vi "Farming robot v2.vi"() -> ()   [LabVIEW 2021]
uses:
  <vilib>/myRIO/Instrument Drivers/Onboard IO/DIO/typedefs/DIO Reference.ctl
  <vilib>/myRIO/Common/Instrument Driver Framework/Utilities/typedefs/myRIO Generic Hardware Reference.ctl
  <vilib>/myRIO/Common/Instrument Driver Framework/Utilities/typedefs/Hardware Version Enum.ctl
  <vilib>/myRIO/Common/Instrument Driver Framework/Utilities/typedefs/myRIO v1.0 Reference.ctl
  <vilib>/myRIO/Common/Instrument Driver Framework/Utilities/typedefs/Generic FPGA Reference.ctl
  <vilib>/myRIO/Common/Instrument Driver Framework/myRIO v1.0/DIO/typedefs/DIO Channels List.ctl
  <vilib>/myRIO/Common/Instrument Driver Framework/myRIO v1.0/DIO/typedefs/DIO Channels Enum.ctl
  <vilib>/userDefined/High Color/nirio_resource_hc.ctl
  <vilib>/myRIO/Instrument Drivers/Onboard IO/PWM/typedefs/PWM Reference.ctl
  <vilib>/myRIO/Common/Instrument Driver Framework/myRIO v1.0/PWM/typedefs/PWM Channels Enum.ctl
  <vilib>/myRIO/Instrument Drivers/Onboard IO/PWM/typedefs/PWM Configuration.ctl
  <vilib>/myRIO/Instrument Drivers/Onboard Devices/Accelerometer/typedefs/Accelerometer Reference.ctl
  <vilib>/myRIO/Common/Instrument Driver Framework/myRIO v1.0/Accelerometer/typedefs/Accelerometer Channels List.ctl
  <vilib>/myRIO/Common/Instrument Driver Framework/myRIO v1.0/Accelerometer/typedefs/Accelerometer Channels Enum.ctl
  <vilib>/myRIO/Common/Instrument Driver Framework/Utilities/vis/Is FPGA Ref Available.vi
  <vilib>/myRIO/Common/Instrument Driver Framework/myRIO v1.0/DIO/vis/myRIO v1.1 Open DIO.vi
  <vilib>/myRIO/Instrument Drivers/Onboard IO/DIO/vis/Write.vi
  <vilib>/myRIO/Common/Instrument Driver Framework/myRIO v1.0/Accelerometer/vis/myRIO v1.1 Open Accelerometer.vi
  <vilib>/myRIO/Instrument Drivers/Onboard Devices/Accelerometer/vis/Read.vi
  <vilib>/myRIO/Common/Instrument Driver Framework/myRIO v1.0/PWM/vis/myRIO v1.1 Open PWM.vi
  <vilib>/myRIO/Instrument Drivers/Onboard IO/PWM/vis/Set Duty Cycle and Frequency.vi
  <vilib>/myRIO/Common/Instrument Driver Framework/Utilities/vis/Validate Channels.vi
  <vilib>/myRIO/Common/Instrument Driver Framework/myRIO v1.0/DIO/vis/myRIO v1.0 Reserve DIO.vi
  <vilib>/myRIO/Common/Instrument Driver Framework/myRIO v1.0/Accelerometer/vis/myRIO v1.0 Reserve Accelerometer.vi
  <vilib>/myRIO/Common/Instrument Driver Framework/myRIO v1.0/PWM/vis/myRIO v1.0 Reserve PWM.vi
  <vilib>/myRIO/Common/Instrument Driver Framework/myRIO v1.0/Resource Manager/vis/myRIO v1.0 Reserve Channel List.vi
  <vilib>/myRIO/Common/Instrument Driver Framework/myRIO v1.0/DIO/vis/myRIO v1.0 Build MUX Configuration DIO.vi
  <vilib>/myRIO/Common/Instrument Driver Framework/myRIO v1.0/Accelerometer/vis/myRIO v1.0 Build MUX Configuration Accelerometer.vi
  <vilib>/myRIO/Common/Instrument Driver Framework/myRIO v1.0/PWM/vis/myRIO v1.0 Build MUX Configuration PWM.vi
  <vilib>/myRIO/Common/Instrument Driver Framework/myRIO v1.0/Resource Manager/vis/myRIO v1.0 Reserve Channel.vi
  <vilib>/myRIO/Common/Instrument Driver Framework/myRIO v1.0/Resource Manager/vis/myRIO v1.0 Unreserve Channel.vi
  <vilib>/myRIO/Common/Instrument Driver Framework/myRIO v1.0/Resource Manager/vis/myRIO v1.0 Create Configuration List.vi
  <vilib>/myRIO/Common/Instrument Driver Framework/myRIO v1.0/Resource Manager/vis/myRIO v1.0 Build Mutex Name.vi
  <vilib>/Utility/VariantDataType/GetNumericInfo.vi
  <vilib>/Utility/error.llb/Error Cluster From Error Code.vi
  <vilib>/myRIO/Common/Instrument Driver Framework/myRIO v1.0/myRIO v1.1 Open.vi
  <vilib>/myRIO/Common/Instrument Driver Framework/Utilities/vis/IO Manager.vi
  <vilib>/myRIO/Common/Instrument Driver Framework/Utilities/vis/Configuration Manager.vi
  <vilib>/myRIO/Common/Instrument Driver Framework/myRIO v1.0/Resource Manager/vis/myRIO v1.0 Configure IO.vi
  <vilib>/myRIO/Common/Instrument Driver Framework/myRIO v1.0/myRIO v1.0 Close.vi
  <vilib>/myRIO/Common/Instrument Driver Framework/myRIO v1.0/DIO/vis/myRIO v1.0 Write DIO.vi
  <vilib>/myRIO/Common/Instrument Driver Framework/myRIO v1.0/PWM/vis/myRIO v1.0 Write PWM.vi
  <vilib>/myRIO/Common/Instrument Driver Framework/myRIO v1.0/Accelerometer/vis/myRIO v1.0 Get Scaling Constant Accelerometer.vi
  <vilib>/myRIO/Common/Instrument Driver Framework/myRIO v1.0/Accelerometer/vis/myRIO v1.0 Read Accelerometer.vi
  <vilib>/myRIO/Express VI/Onboard Devices/LED/LED Express VI.xnode
  <vilib>/myRIO/Instrument Drivers/Onboard IO/DIO/vis/myRIO DIO Open.xnode
  <vilib>/myRIO/Express VI/Onboard IO/DO/DO Express VI.xnode
  <vilib>/myRIO/Express VI/Onboard IO/PWM/PWM Express VI.xnode
  <vilib>/myRIO/Instrument Drivers/Onboard IO/PWM/vis/myRIO PWM Open.xnode
  <vilib>/myRIO/Express VI/Onboard Devices/Accelerometer/Accelerometer Express VI.xnode
  <vilib>/myRIO/Instrument Drivers/Onboard Devices/Accelerometer/vis/myRIO Accelerometer Open.xnode
  <vilib>/myRIO/Instrument Drivers/Onboard IO/DIO/DIO.lvlib
  <vilib>/myRIO/Instrument Drivers/Onboard Devices/Accelerometer/Accelerometer.lvlib
  <vilib>/myRIO/Instrument Drivers/Onboard IO/PWM/PWM.lvlib
  <vilib>/Analysis/NI_AALPro.lvlib
panel:
  out "pulse width 2":dbl
  out "Angle 2":dbl
  out "State":T1(ring)
  out "pulse width 1":dbl
  out "Angle 1":dbl
  in  "Start Farming":bool
  out "Watering":bool
  out "Seeding\nUp":bool
  out "Seeding\nDown":bool
  out "Switching\nMode":bool
  out "Drill Up":bool
  out "Drill Down":bool
  out "Intialize":bool
  out "Message":string
  in  "stop":bool
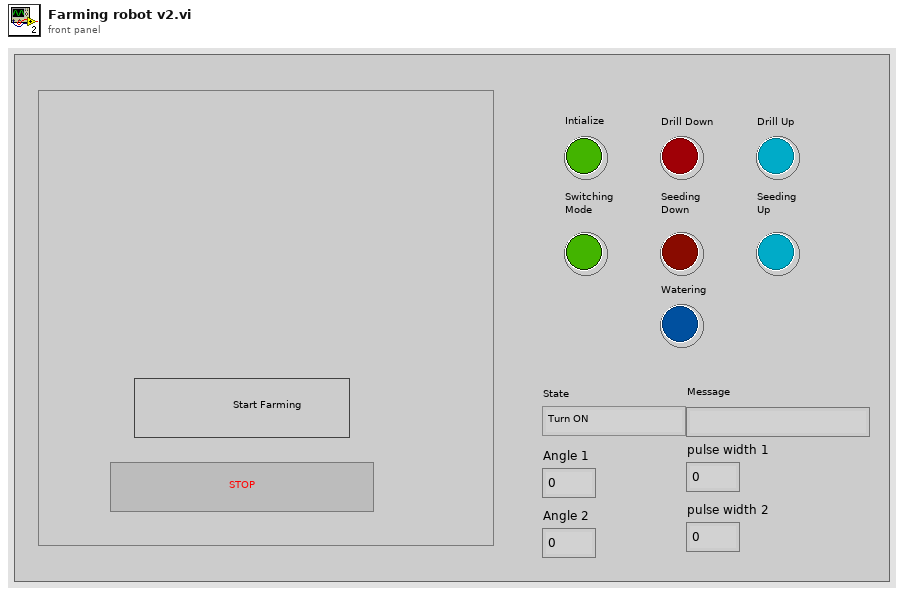
[diagram p1: front panel]
types:
  T1 = enum16{"Turn ON", "IDLE", "Start Farming", "Drive", "Drilling", "Seeding", "Watering", "Filling", "Fell Off", "Stop"}
  T2 = typedef "DIO.lvlib/DIO Reference.ctl" = cluster{"myRIO Reference":T3, "DIO Channels List":T7}
  T3 = typedef "myRIO Generic Hardware Reference.ctl" = cluster{"myRIO Model":T4, "myRIO Hardware Reference":T5}
  T4 = typedef "Hardware Version Enum.ctl" = enum16{"Unknown", "myRIO-1900", "myRIO-1950", "roboRIO", "NI ELVIS RIO CM", "ELVIS III"}
  T5 = typedef "myRIO v1.0 Reference.ctl" = cluster{"Generic FPGA Reference":T6, "Allow multiple opens":bool}
  T6 = typedef "Generic FPGA Reference.ctl" = refnum<k20>
  T7 = typedef "DIO Channels List.ctl" = T8[]
  T8 = typedef "DIO Channels Enum.ctl" = enum16{"Not Connected", "C/DIO0", "C/DIO1", "C/DIO2", "C/DIO3", "C/DIO4", "C/DIO5", "C/DIO6", "C/DIO7", "A/DIO0", "A/DIO1", "A/DIO2", "A/DIO3", "A/DIO4", "A/DIO5", "A/DIO6", "A/DIO7", "A/DIO8", "A/DIO9", "A/DIO10", "A/DIO11", "A/DIO12", "A/DIO13", "A/DIO14", "A/DIO15", "A/DIO16", "A/DIO17", "A/DIO18", "A/DIO19", "B/DIO0", "B/DIO1", "B/DIO2", "B/DIO3", "B/DIO4", "B/DIO5", "B/DIO6", "B/DIO7", "B/DIO8", "B/DIO9", "B/DIO10", "B/DIO11", "B/DIO12", "B/DIO13", "B/DIO14", "B/DIO15", "B/DIO16", "B/DIO17", "B/DIO18", "B/DIO19", "LED0", "LED1", "LED2", "LED3", "Button0", "DIO/DIO0", "DIO/DIO1", "DIO/DIO2", "DIO/DIO3", "DIO/DIO4", "DIO/DIO5", "DIO/DIO6", "DIO/DIO7", "DIO/DIO8", "DIO/DIO9", "SPI/CS0", "SPI/CS1", "SPI/CS2", "SPI/CS3", "LED RADIO (Green)", "LED RADIO (Red)", "LED COMM (Green)", "LED COMM (Red)", "LED MODE (Green)", "LED MODE (Red)"}
  T9 = typedef "nirio_resource_hc.ctl" = tag
  T10 = typedef "PWM.lvlib/PWM Reference.ctl" = cluster{"myRIO Reference":T3, "PWM Channels Enum":T11, "PWM Configuration":T12}
  T11 = typedef "PWM Channels Enum.ctl" = enum16{"Not Connected", "C/PWM0", "C/PWM1", "A/PWM0", "A/PWM1", "A/PWM2", "A/PWM3", "A/PWM4", "A/PWM5", "A/PWM6", "A/PWM7", "A/PWM8", "A/PWM9", "A/PWM10", "A/PWM11", "A/PWM12", "A/PWM13", "A/PWM14", "A/PWM15", "A/PWM16", "A/PWM17", "A/PWM18", "A/PWM19", "B/PWM0", "B/PWM1", "B/PWM2", "B/PWM3", "B/PWM4", "B/PWM5", "B/PWM6", "B/PWM7", "B/PWM8", "B/PWM9", "B/PWM10", "B/PWM11", "B/PWM12", "B/PWM13", "B/PWM14", "B/PWM15", "B/PWM16", "B/PWM17", "B/PWM18", "B/PWM19", "PWM/PWM0", "PWM/PWM1", "PWM/PWM2", "PWM/PWM3", "PWM/PWM4", "PWM/PWM5", "PWM/PWM6", "PWM/PWM7", "PWM/PWM8", "PWM/PWM9"}
  T12 = typedef "PWM.lvlib/PWM Configuration.ctl" = cluster{"Frequency":dbl, "Duty Cycle":dbl}
  T13 = typedef "Accelerometer.lvlib/Accelerometer Reference.ctl" = cluster{"myRIO Reference":T3, "Accelerometer Channels List":T14, "LSB Weight":dbl}
  T14 = typedef "Accelerometer Channels List.ctl" = T15[]
  T15 = typedef "Accelerometer Channels Enum.ctl" = enum16{"Not Connected", "X-Axis", "Y-Axis", "Z-Axis"}
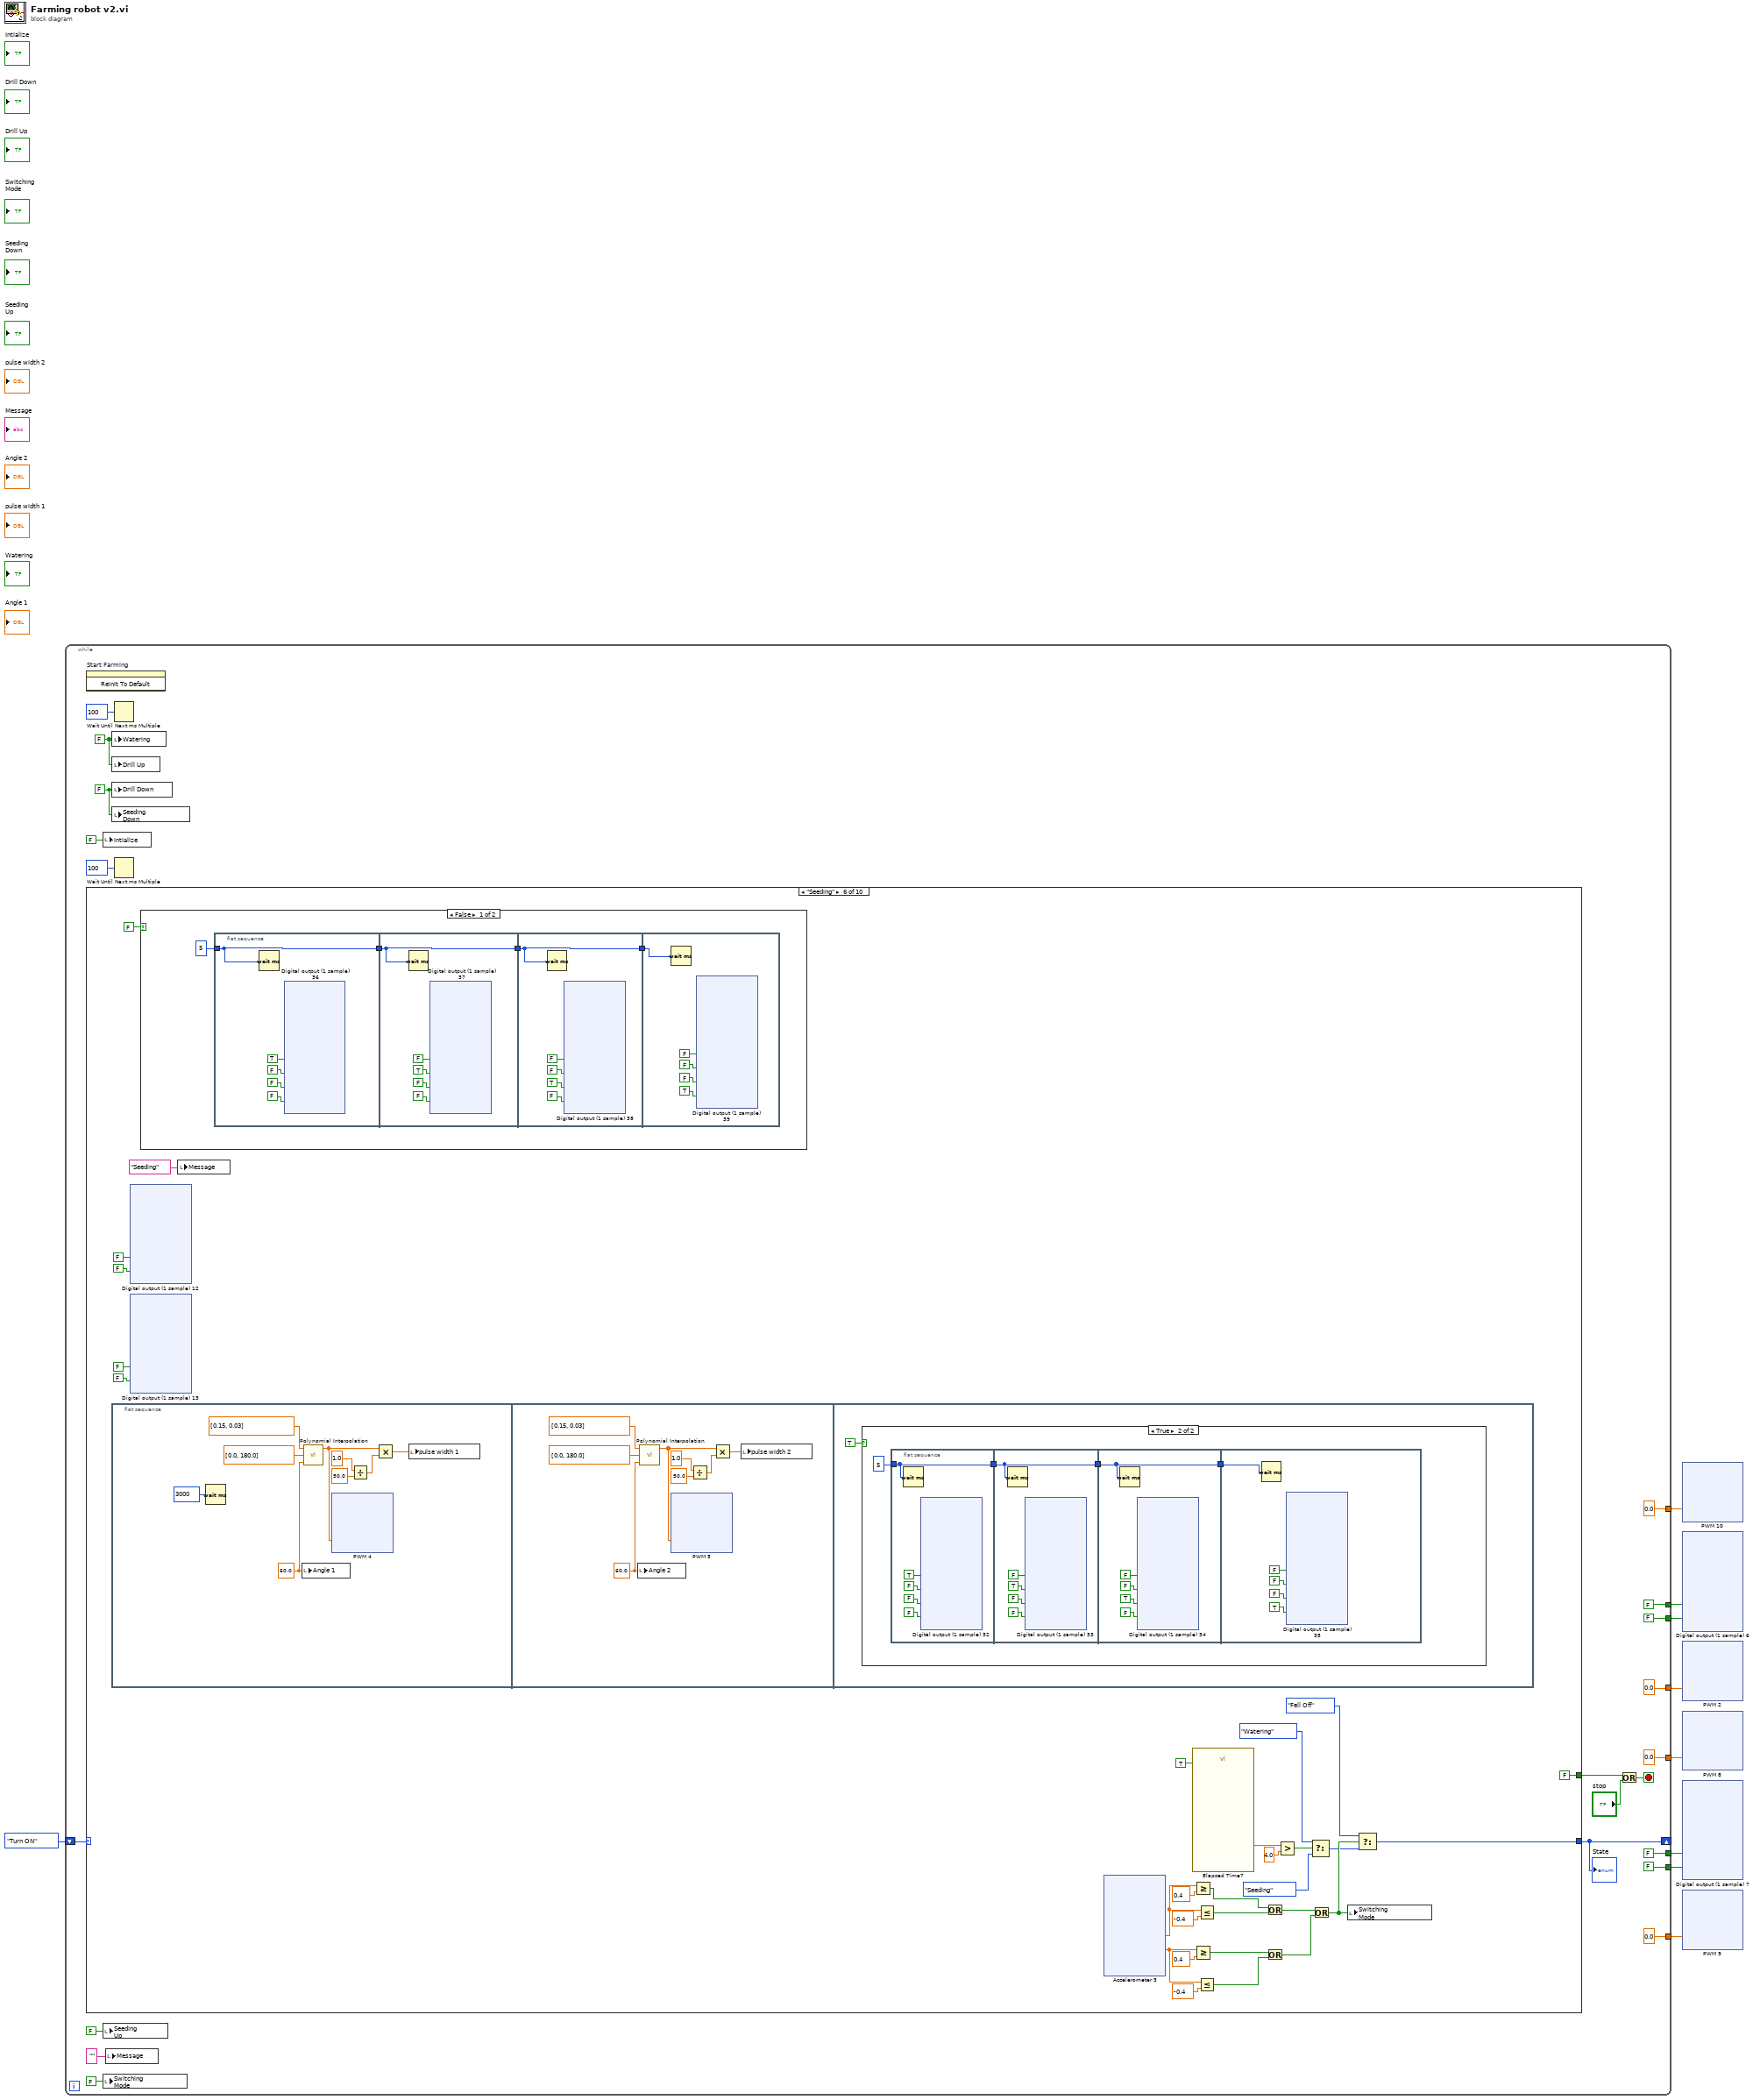
[diagram p0: block diagram]
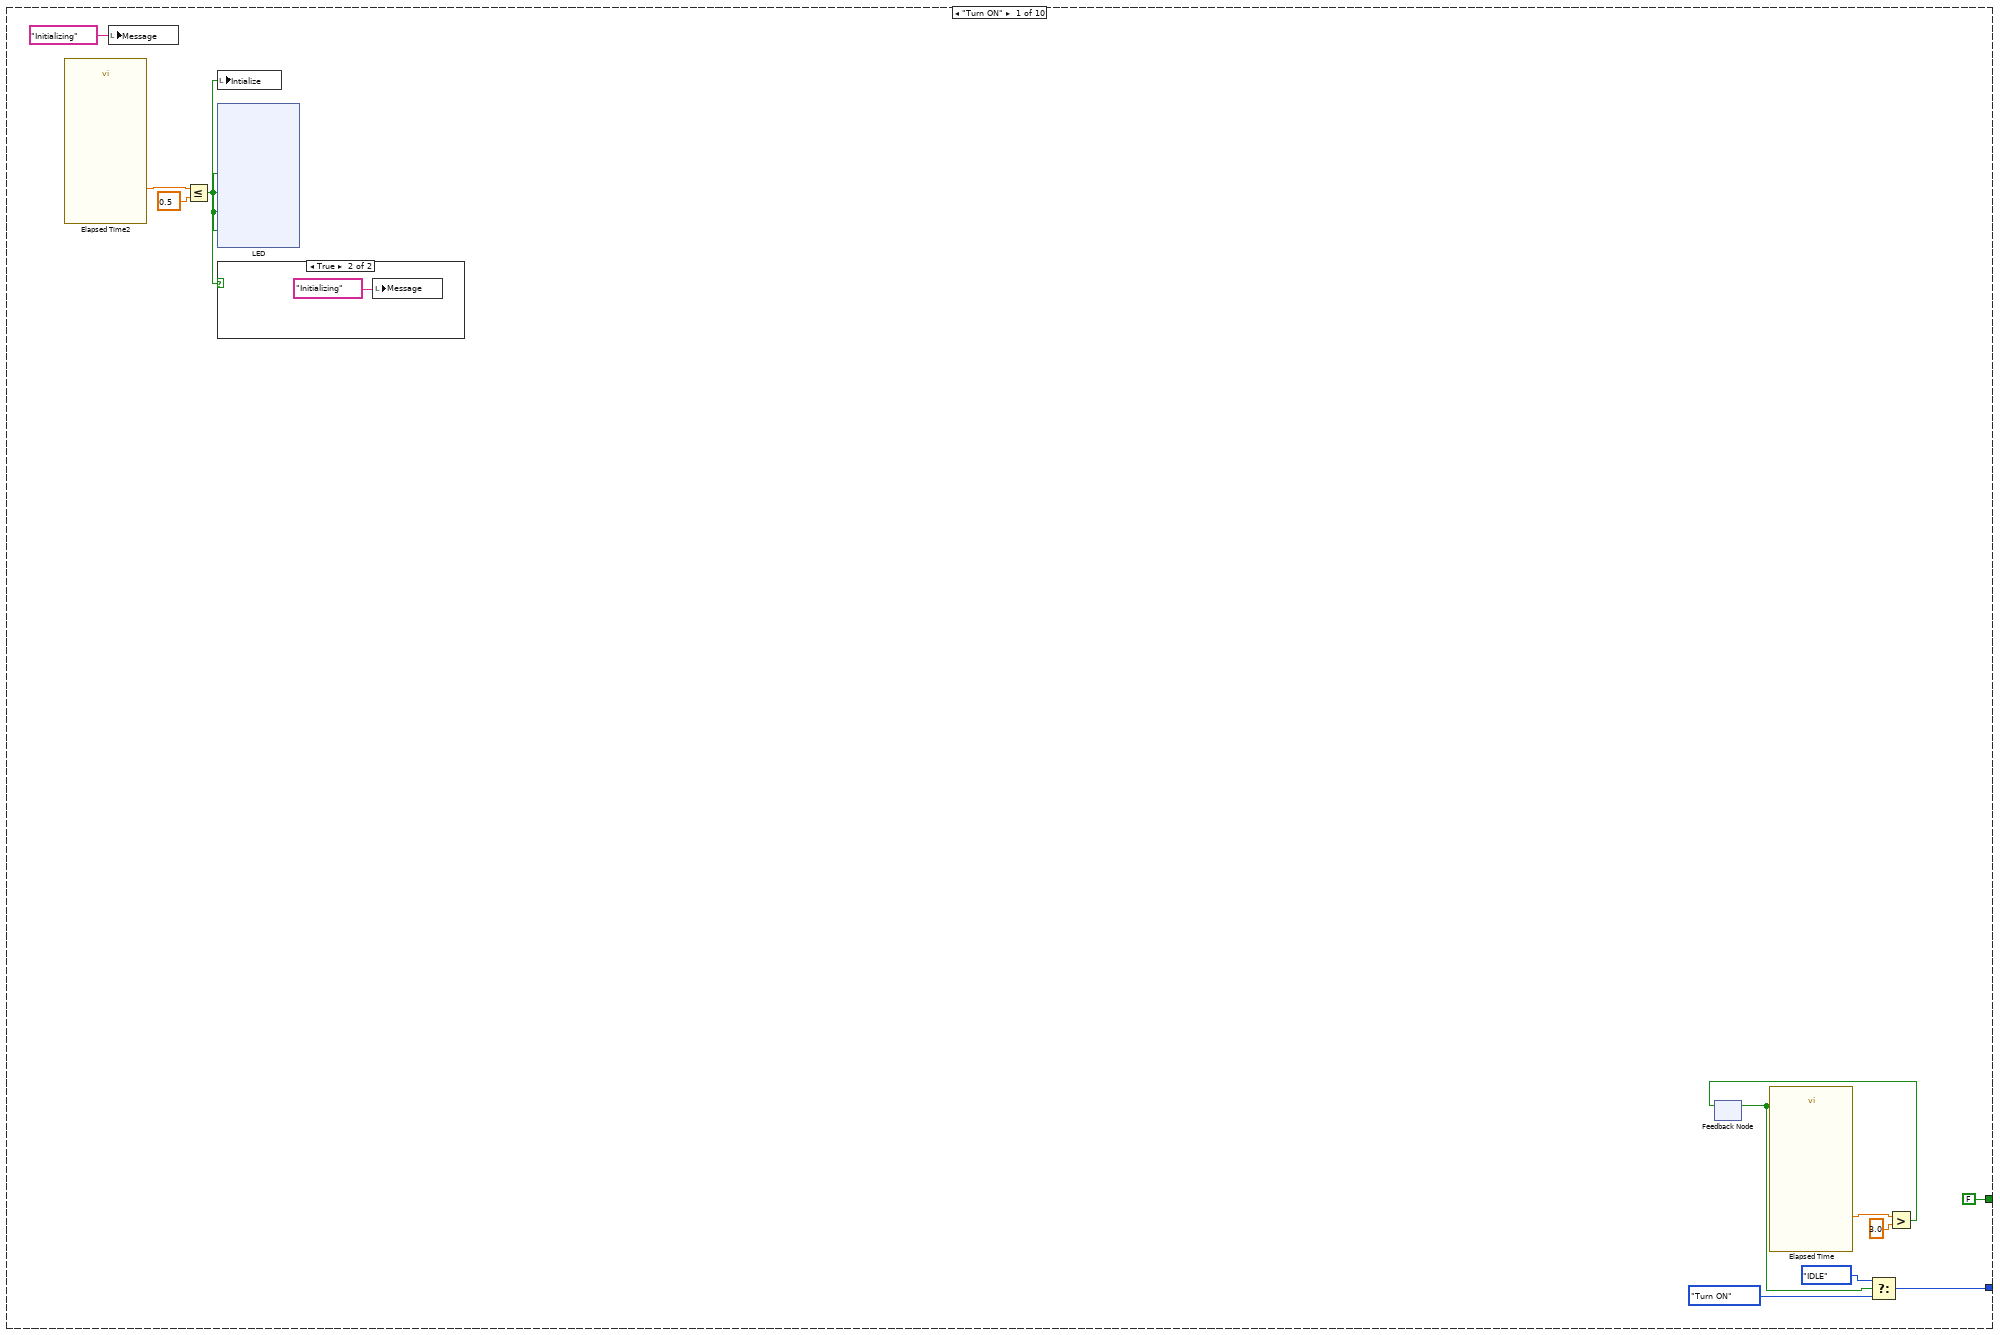
[diagram p2: hidden frame]
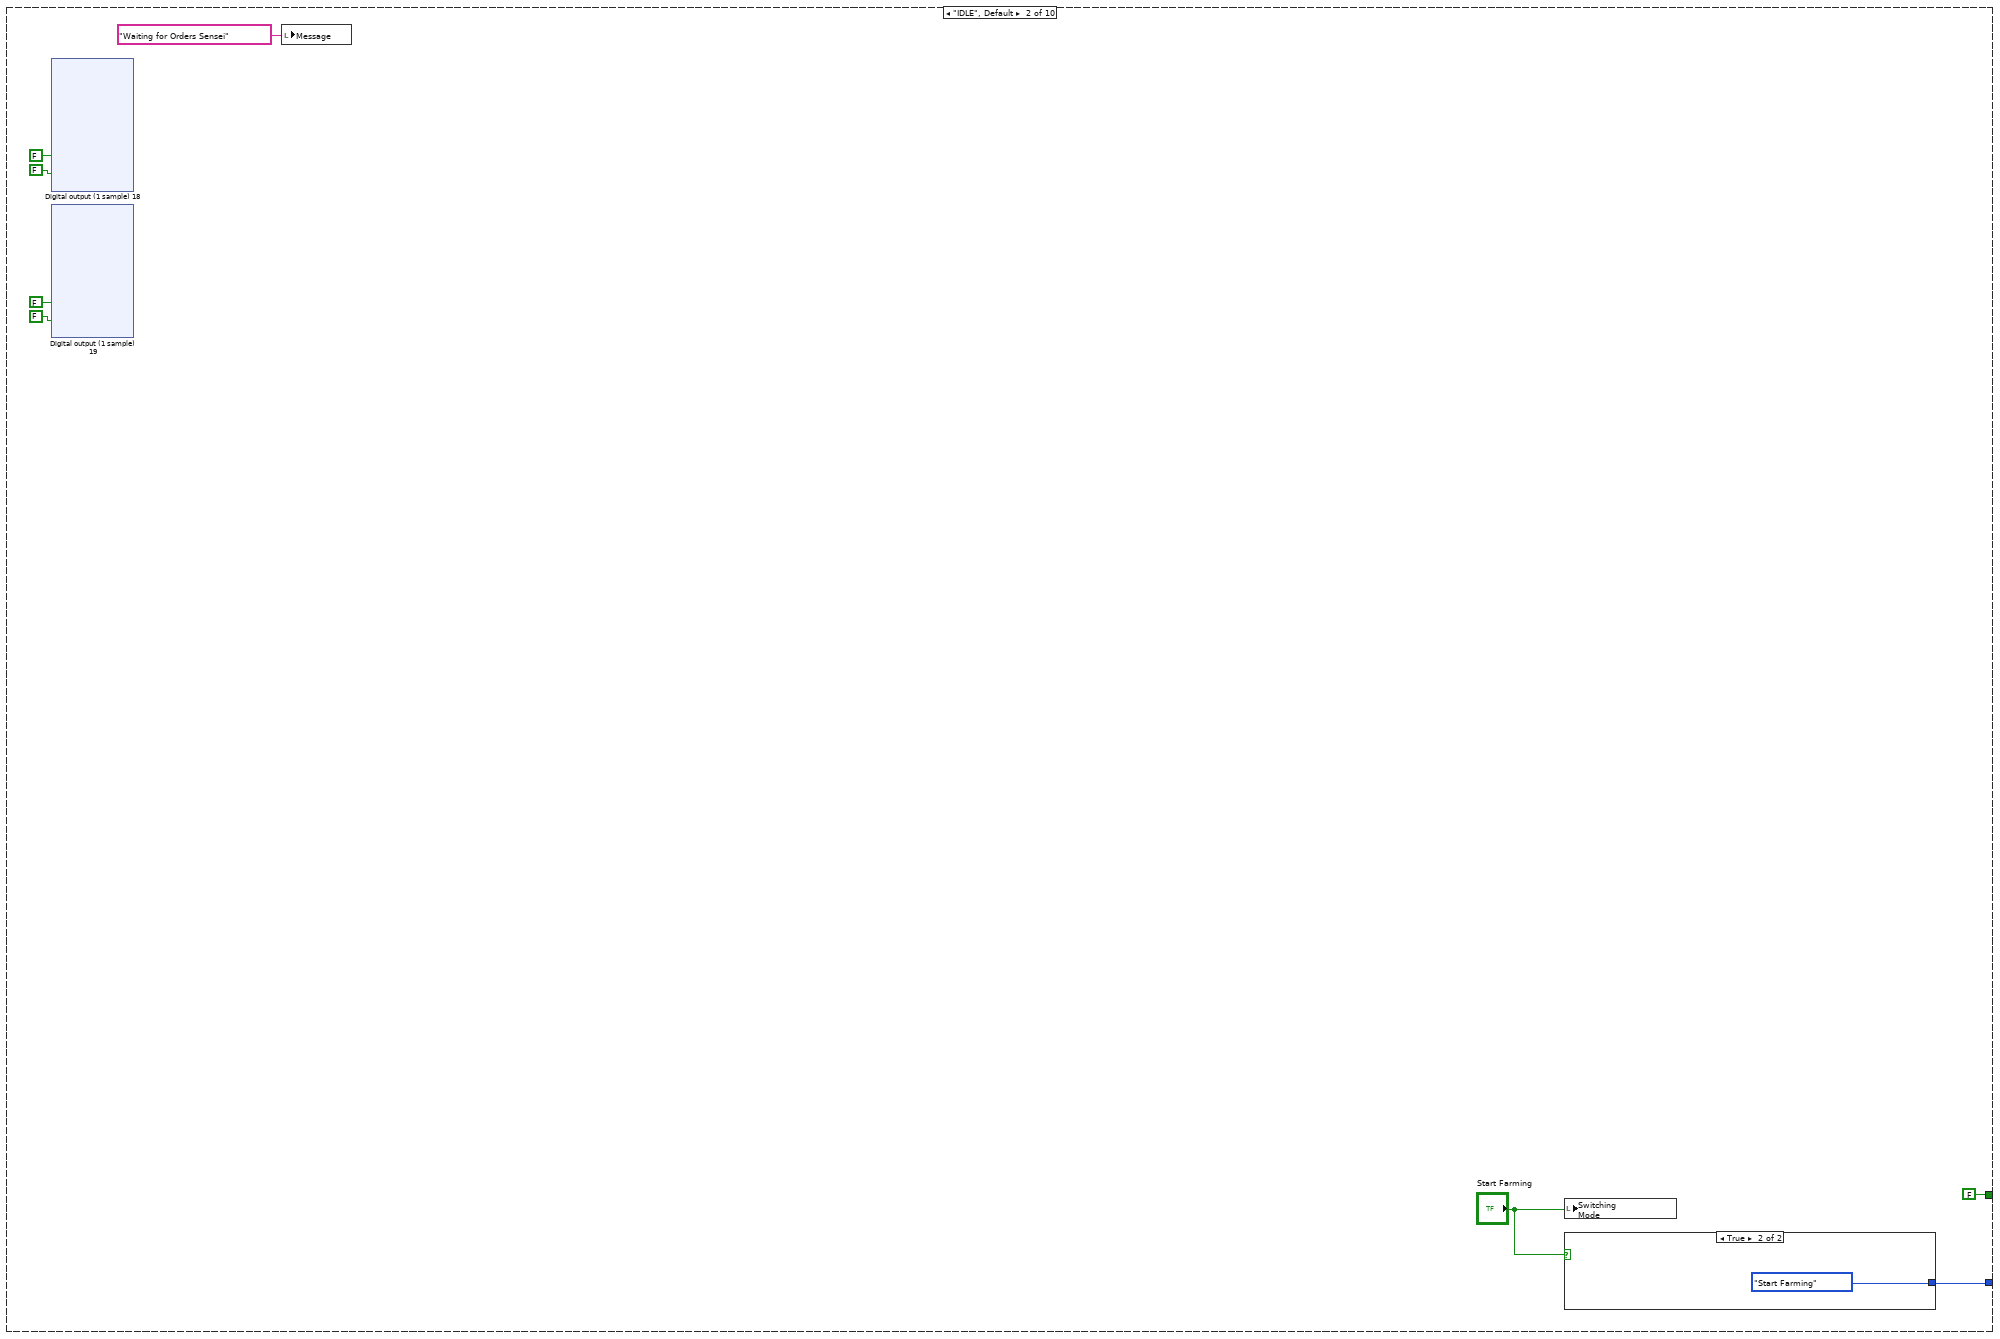
[diagram p4: hidden frame]
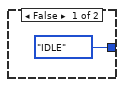
[diagram p5: hidden frame]
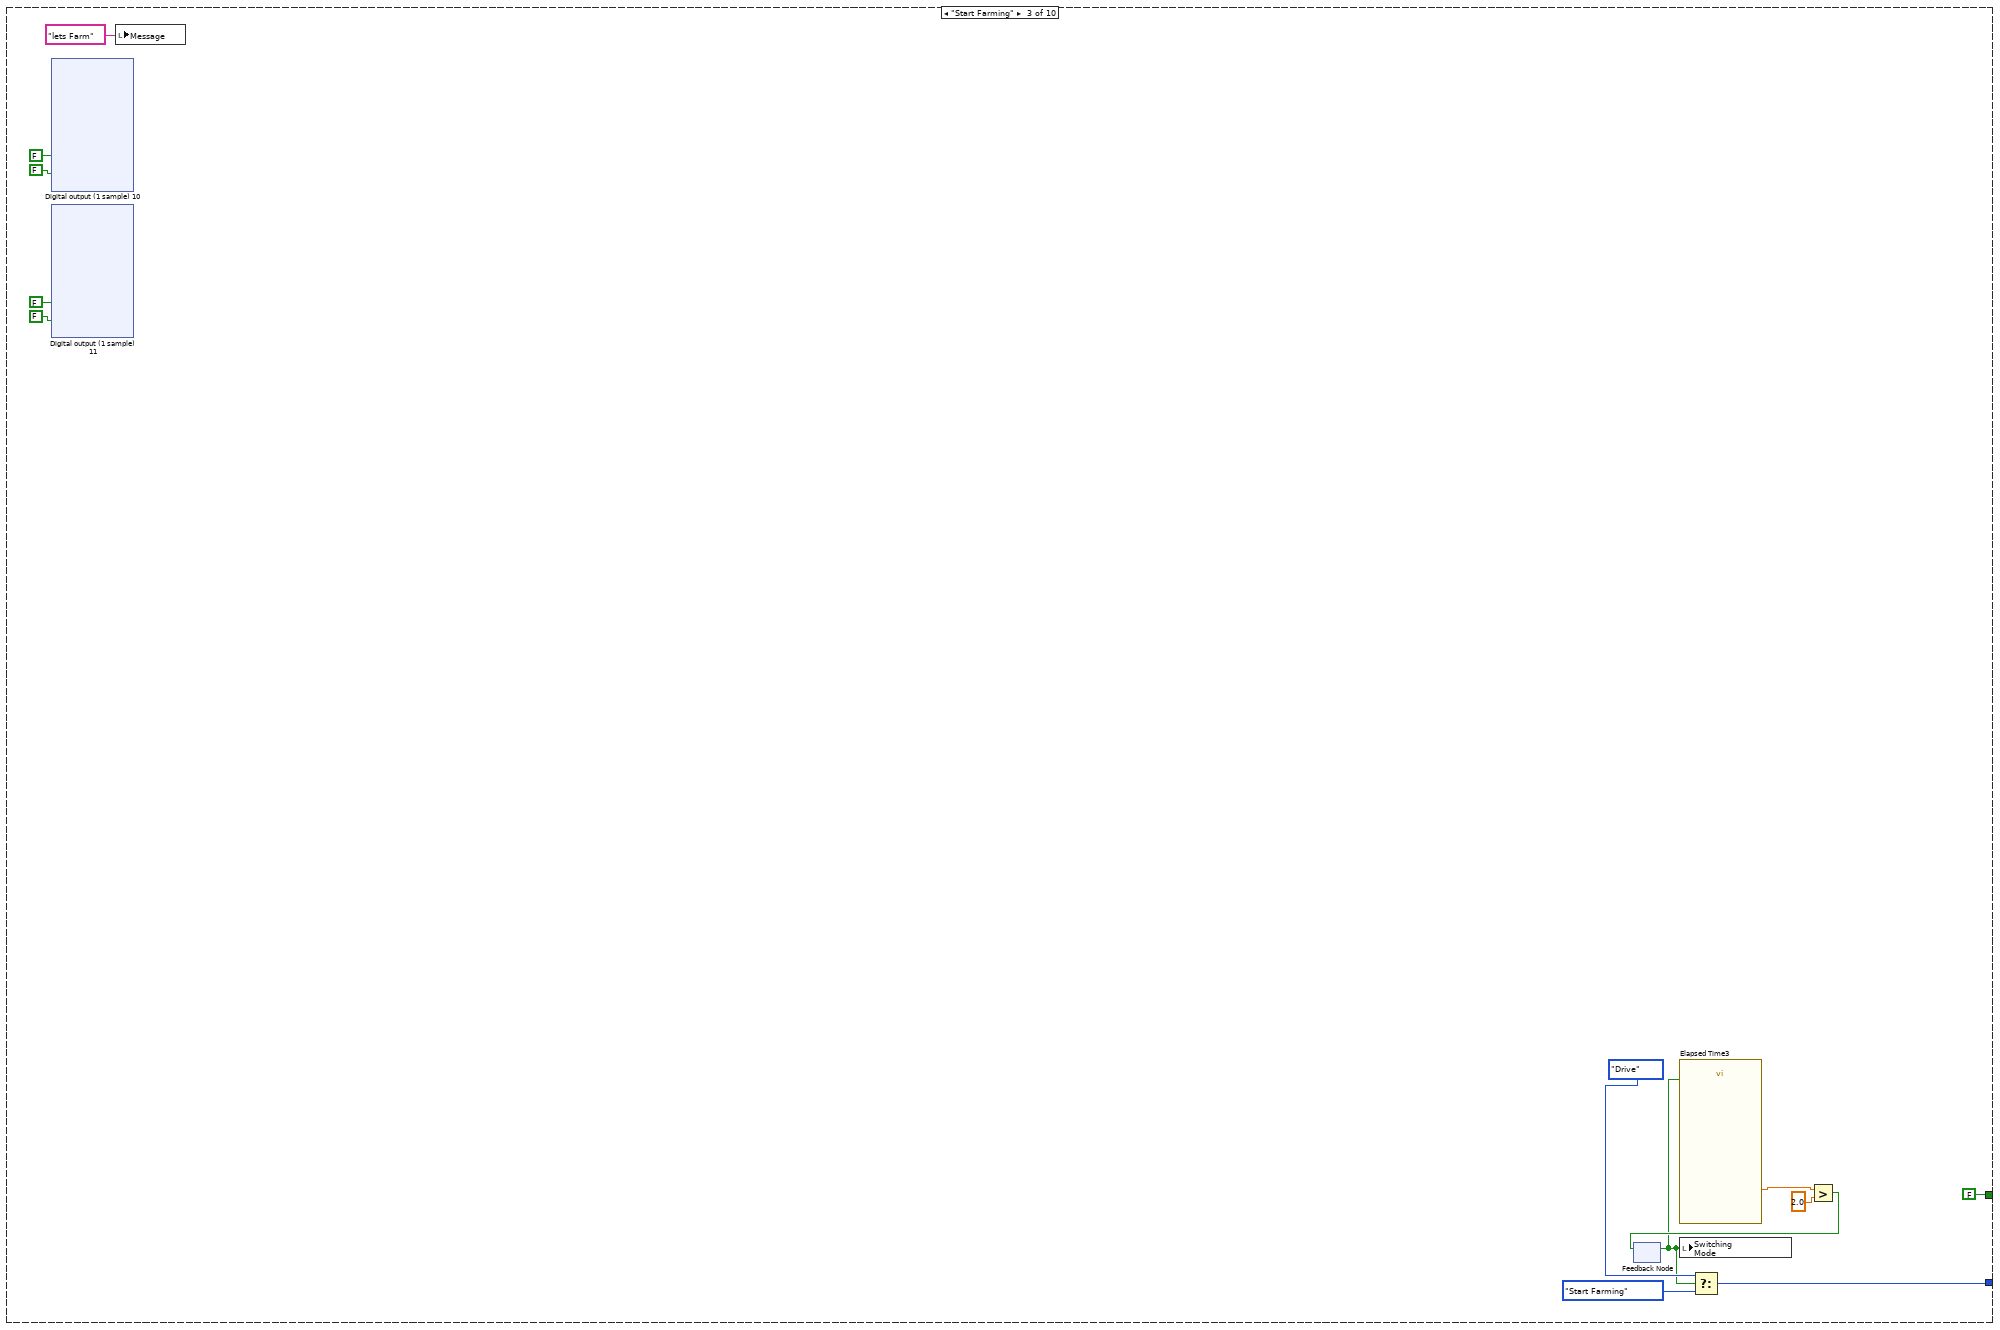
[diagram p6: hidden frame]
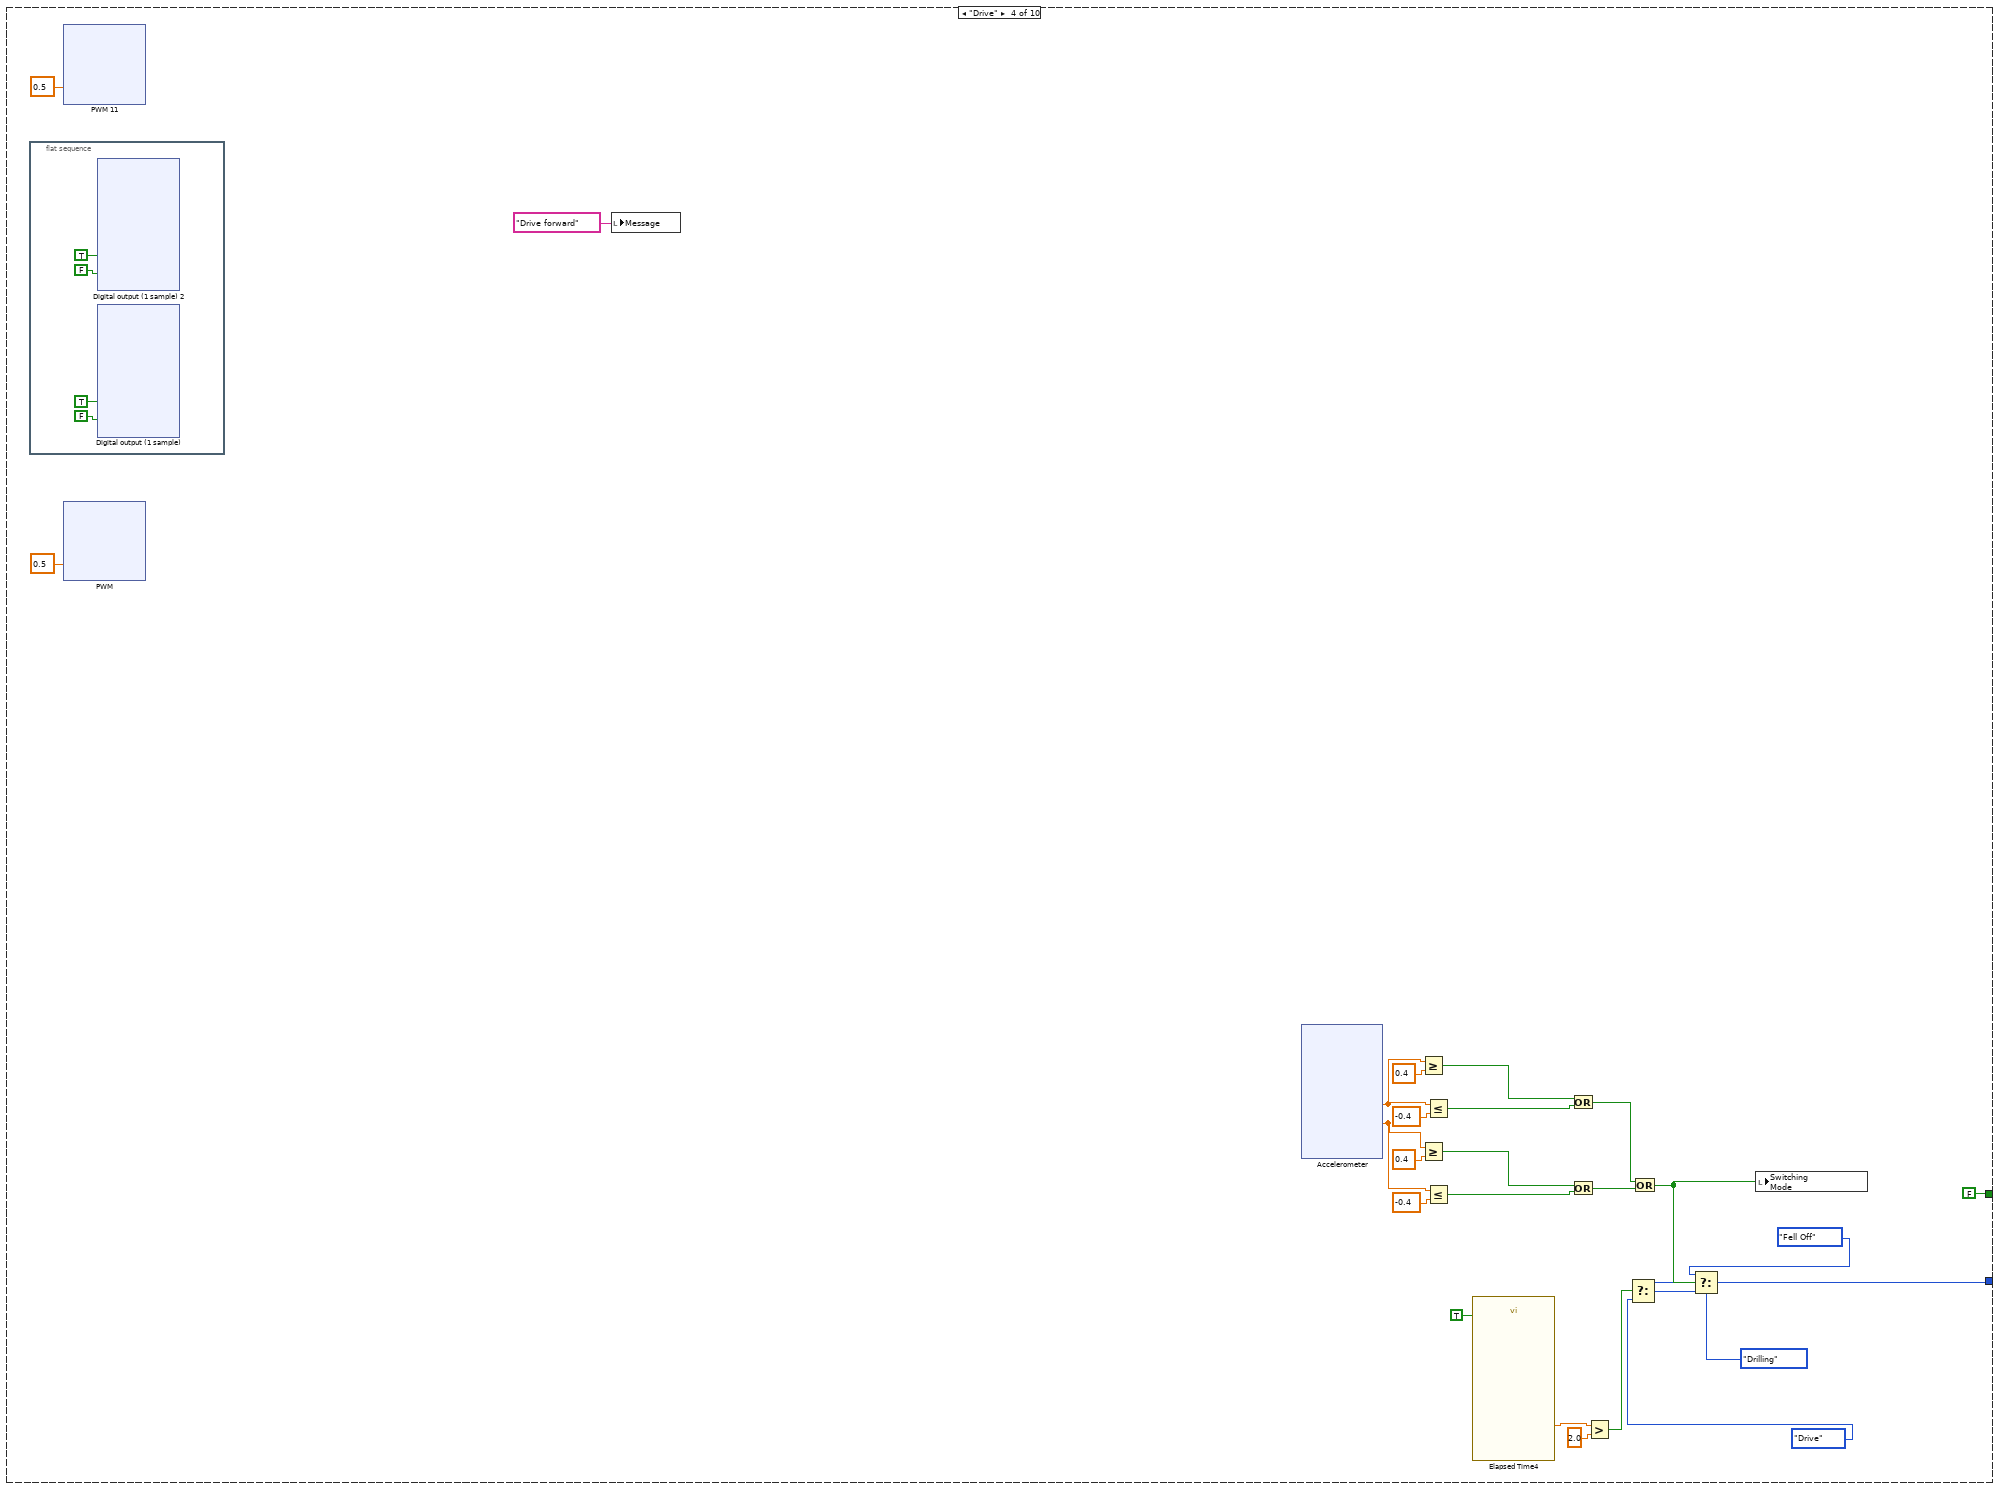
[diagram p7: hidden frame]
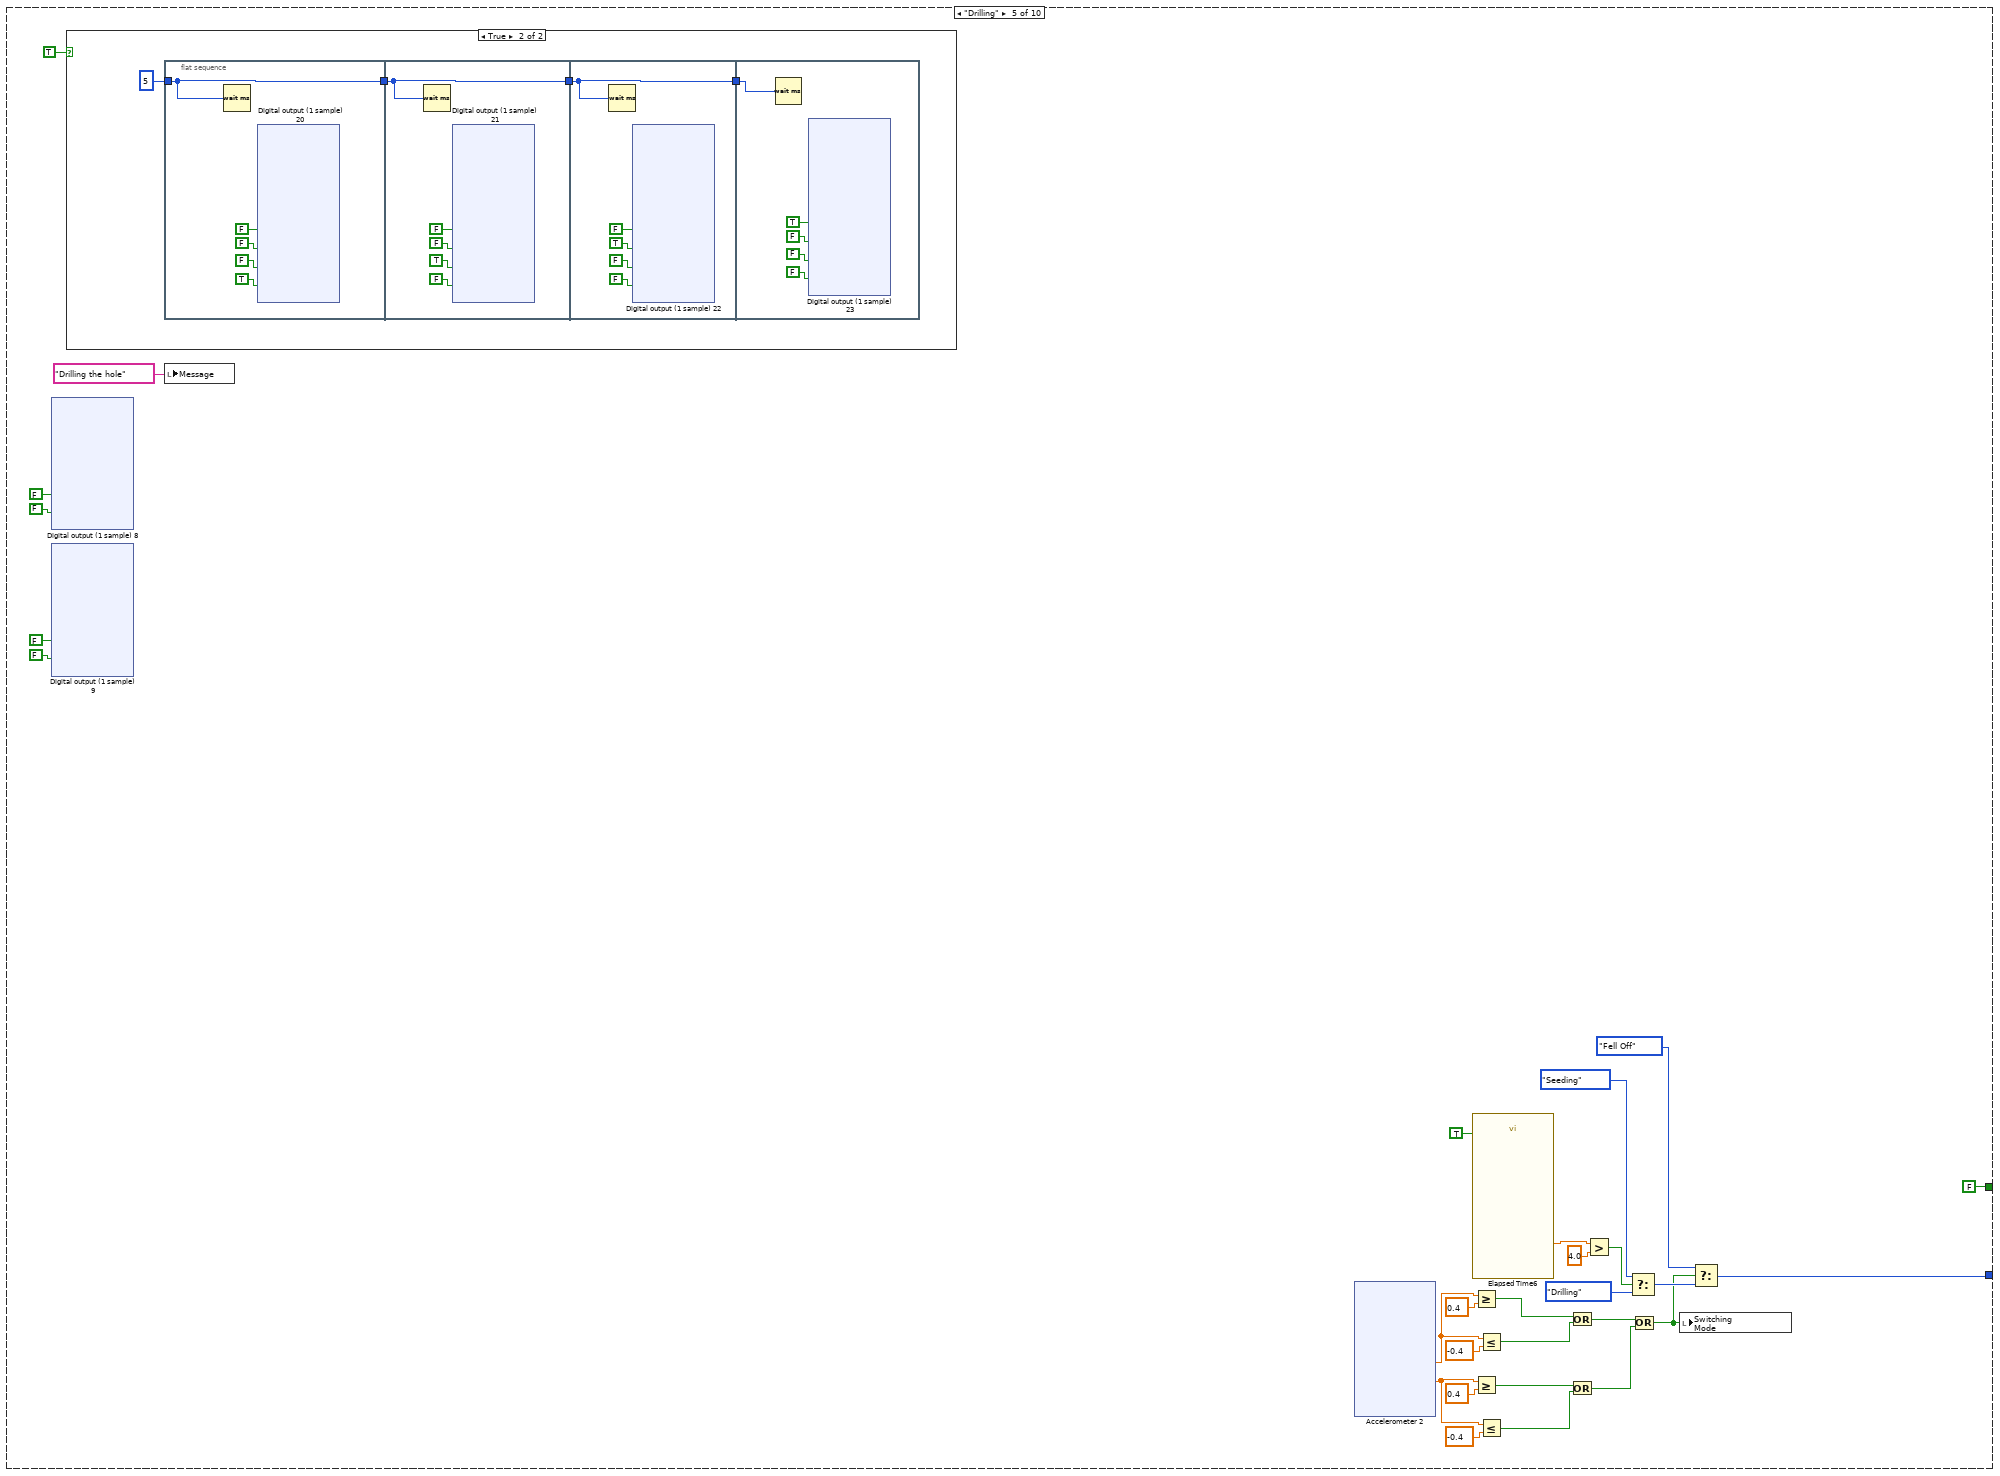
[diagram p8: hidden frame]
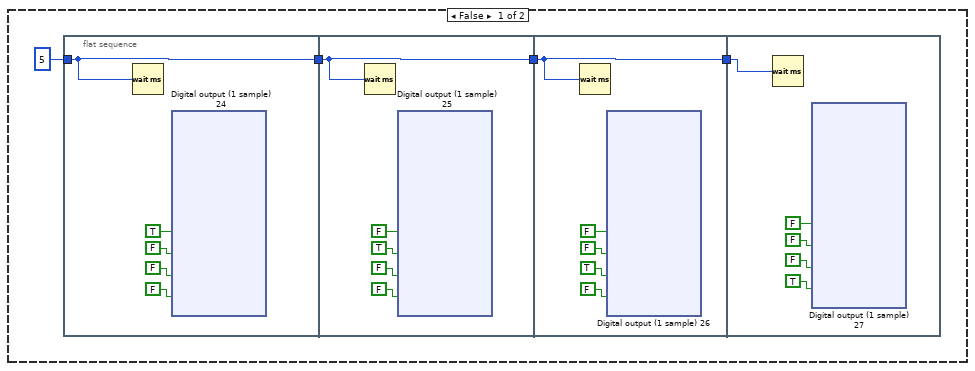
[diagram p9: hidden frame]
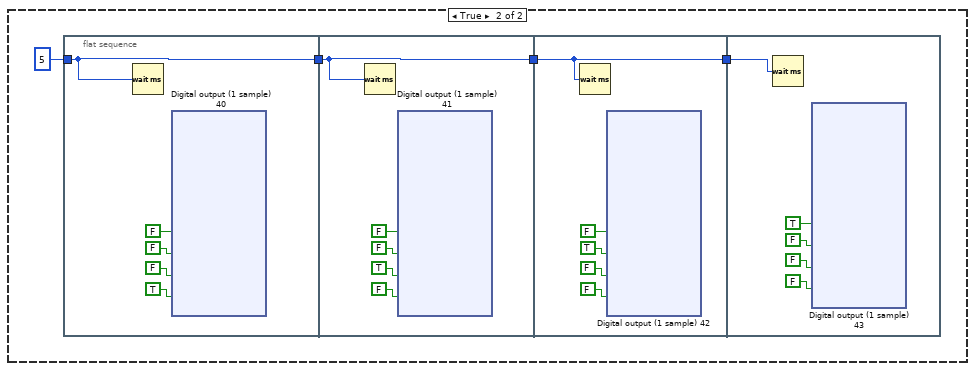
[diagram p10: hidden frame]
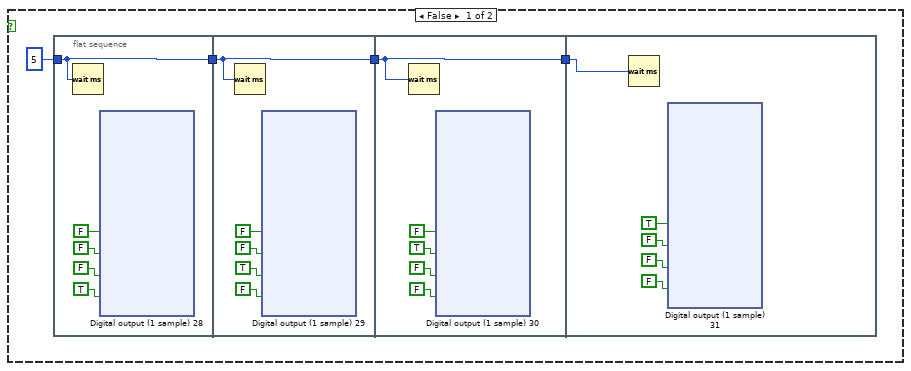
[diagram p11: hidden frame]
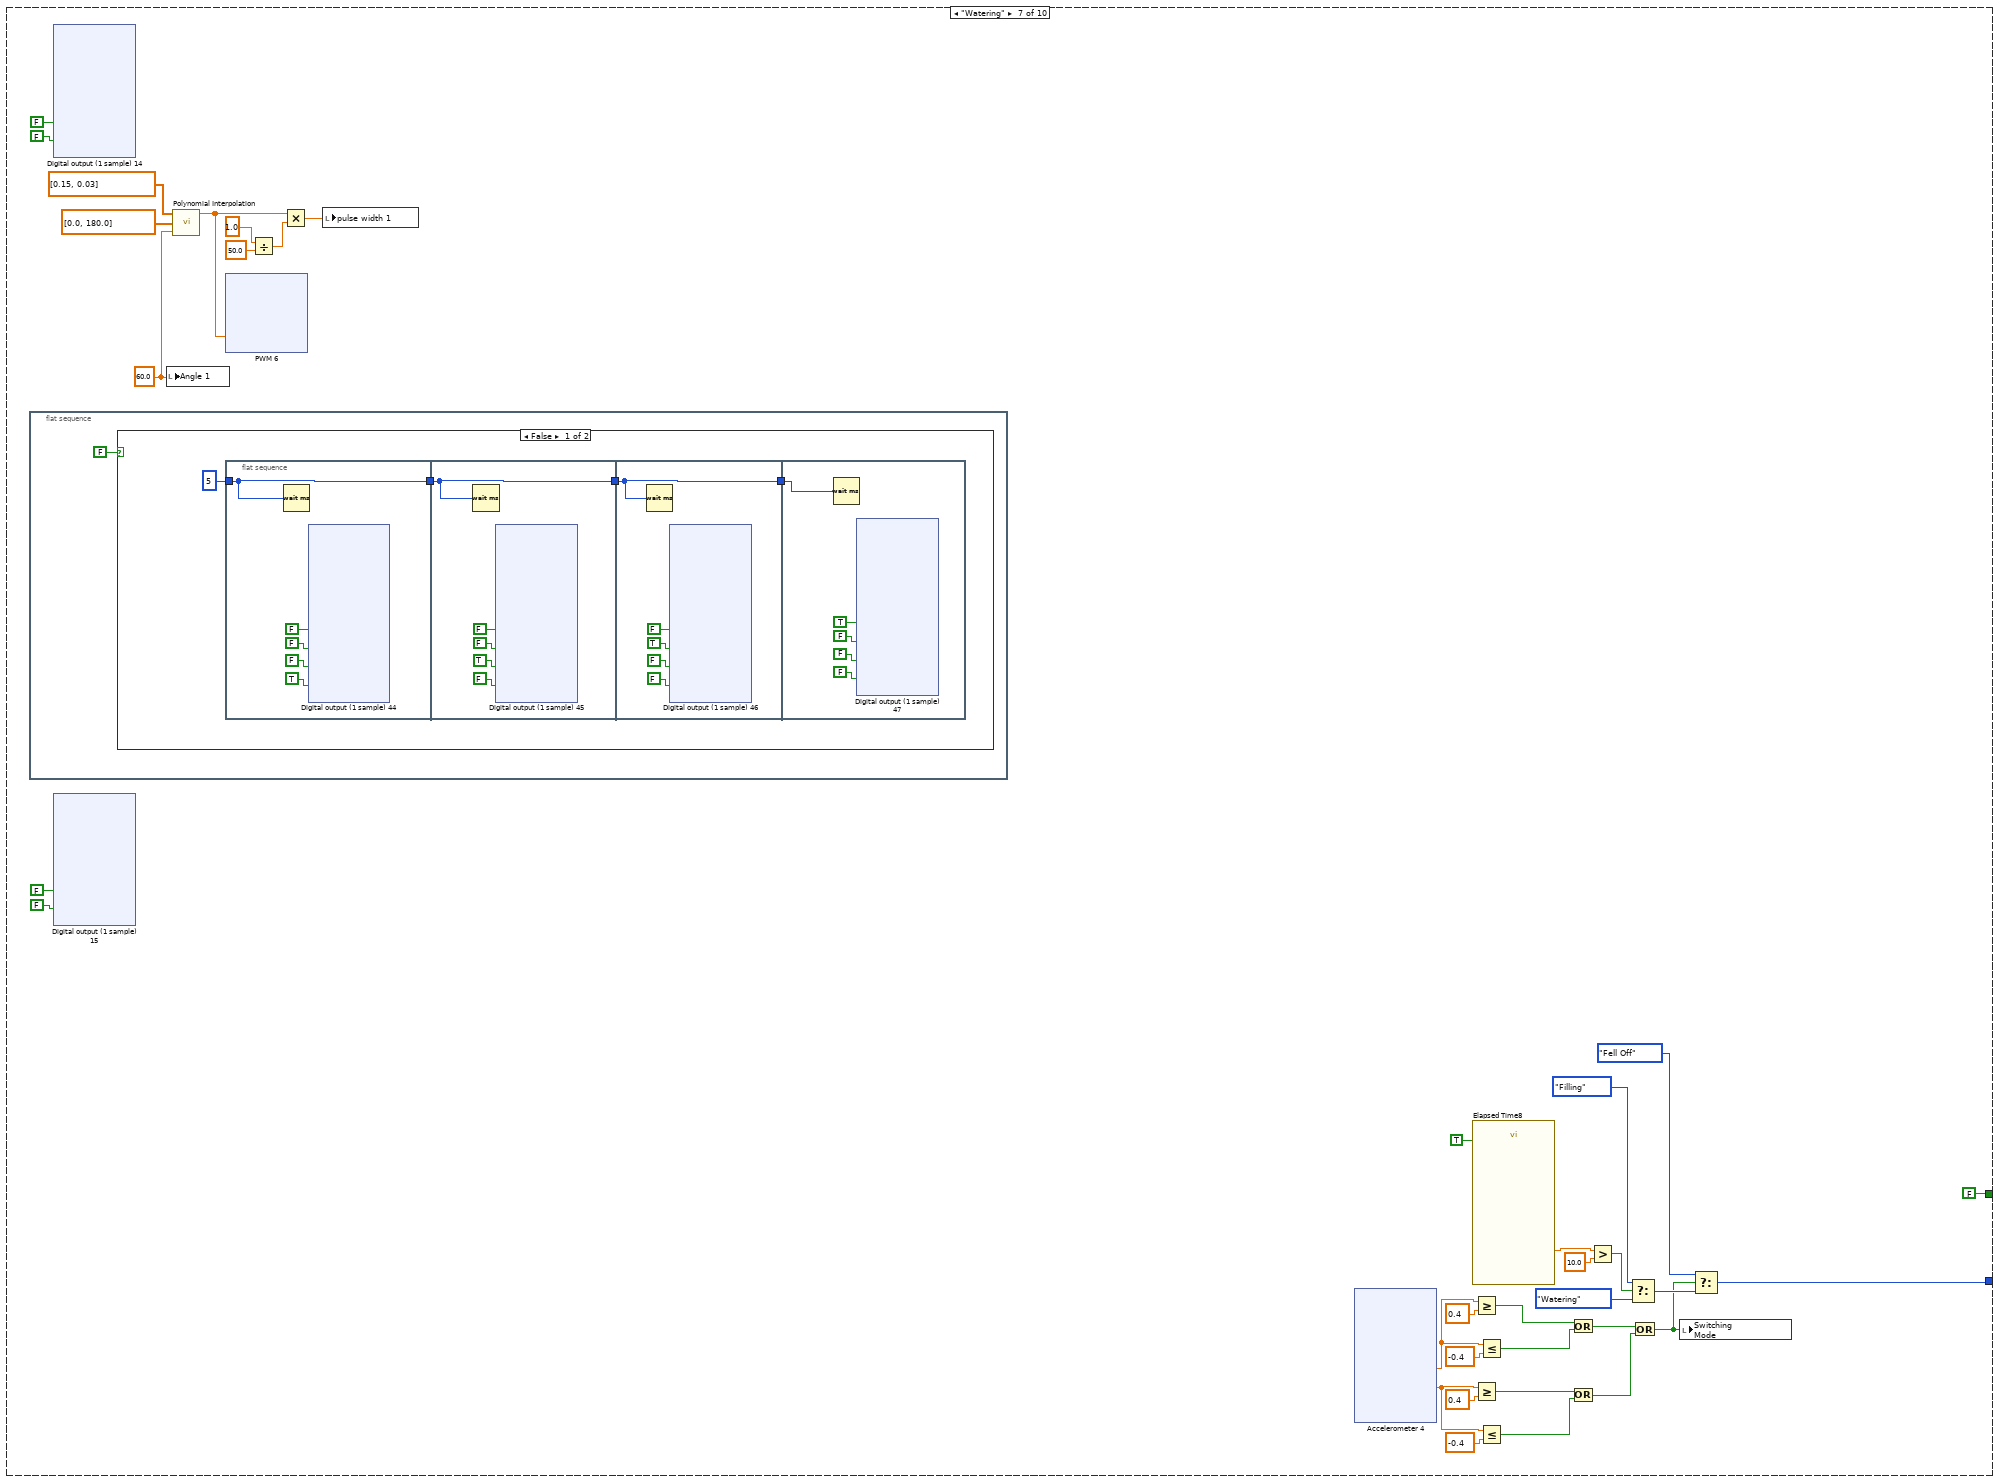
[diagram p12: hidden frame]
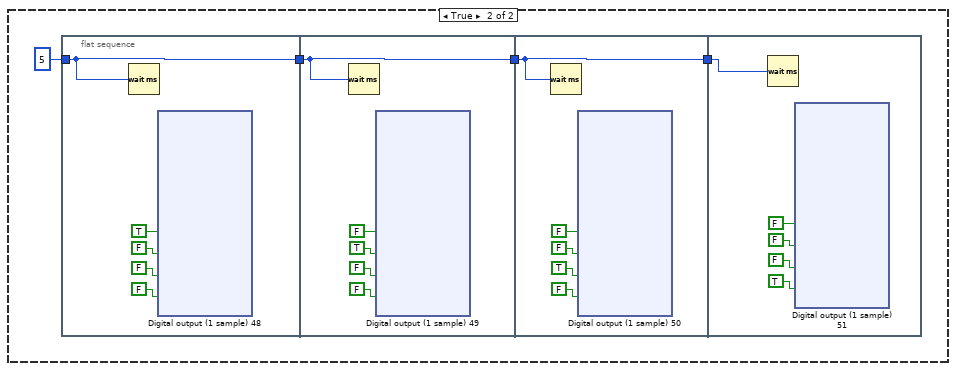
[diagram p13: hidden frame]
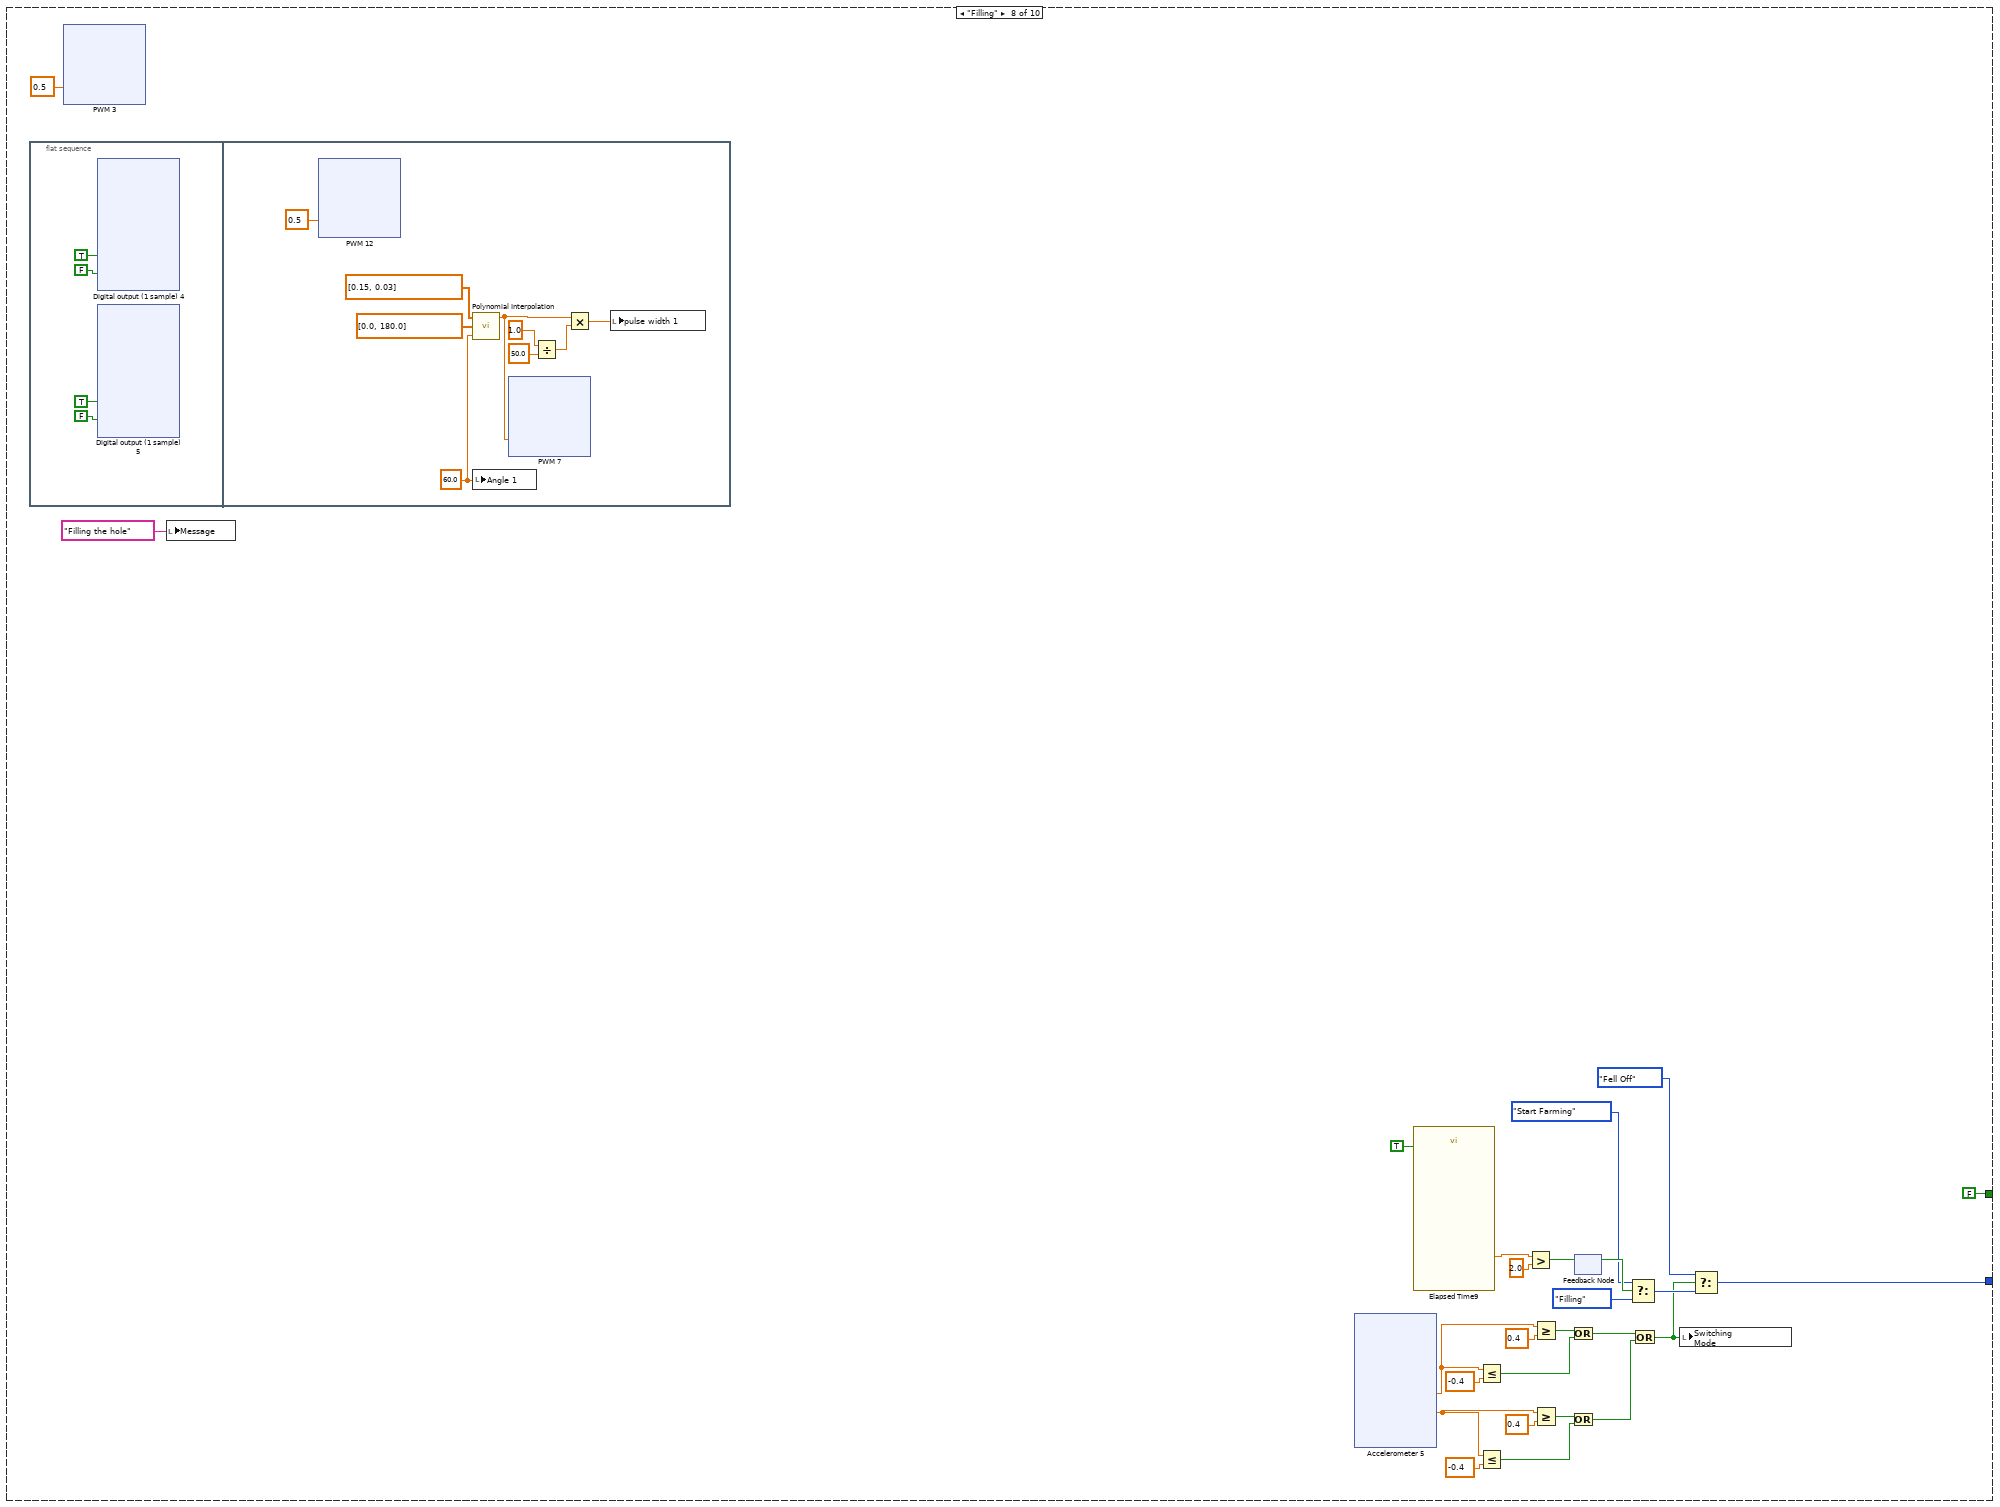
[diagram p14: hidden frame]
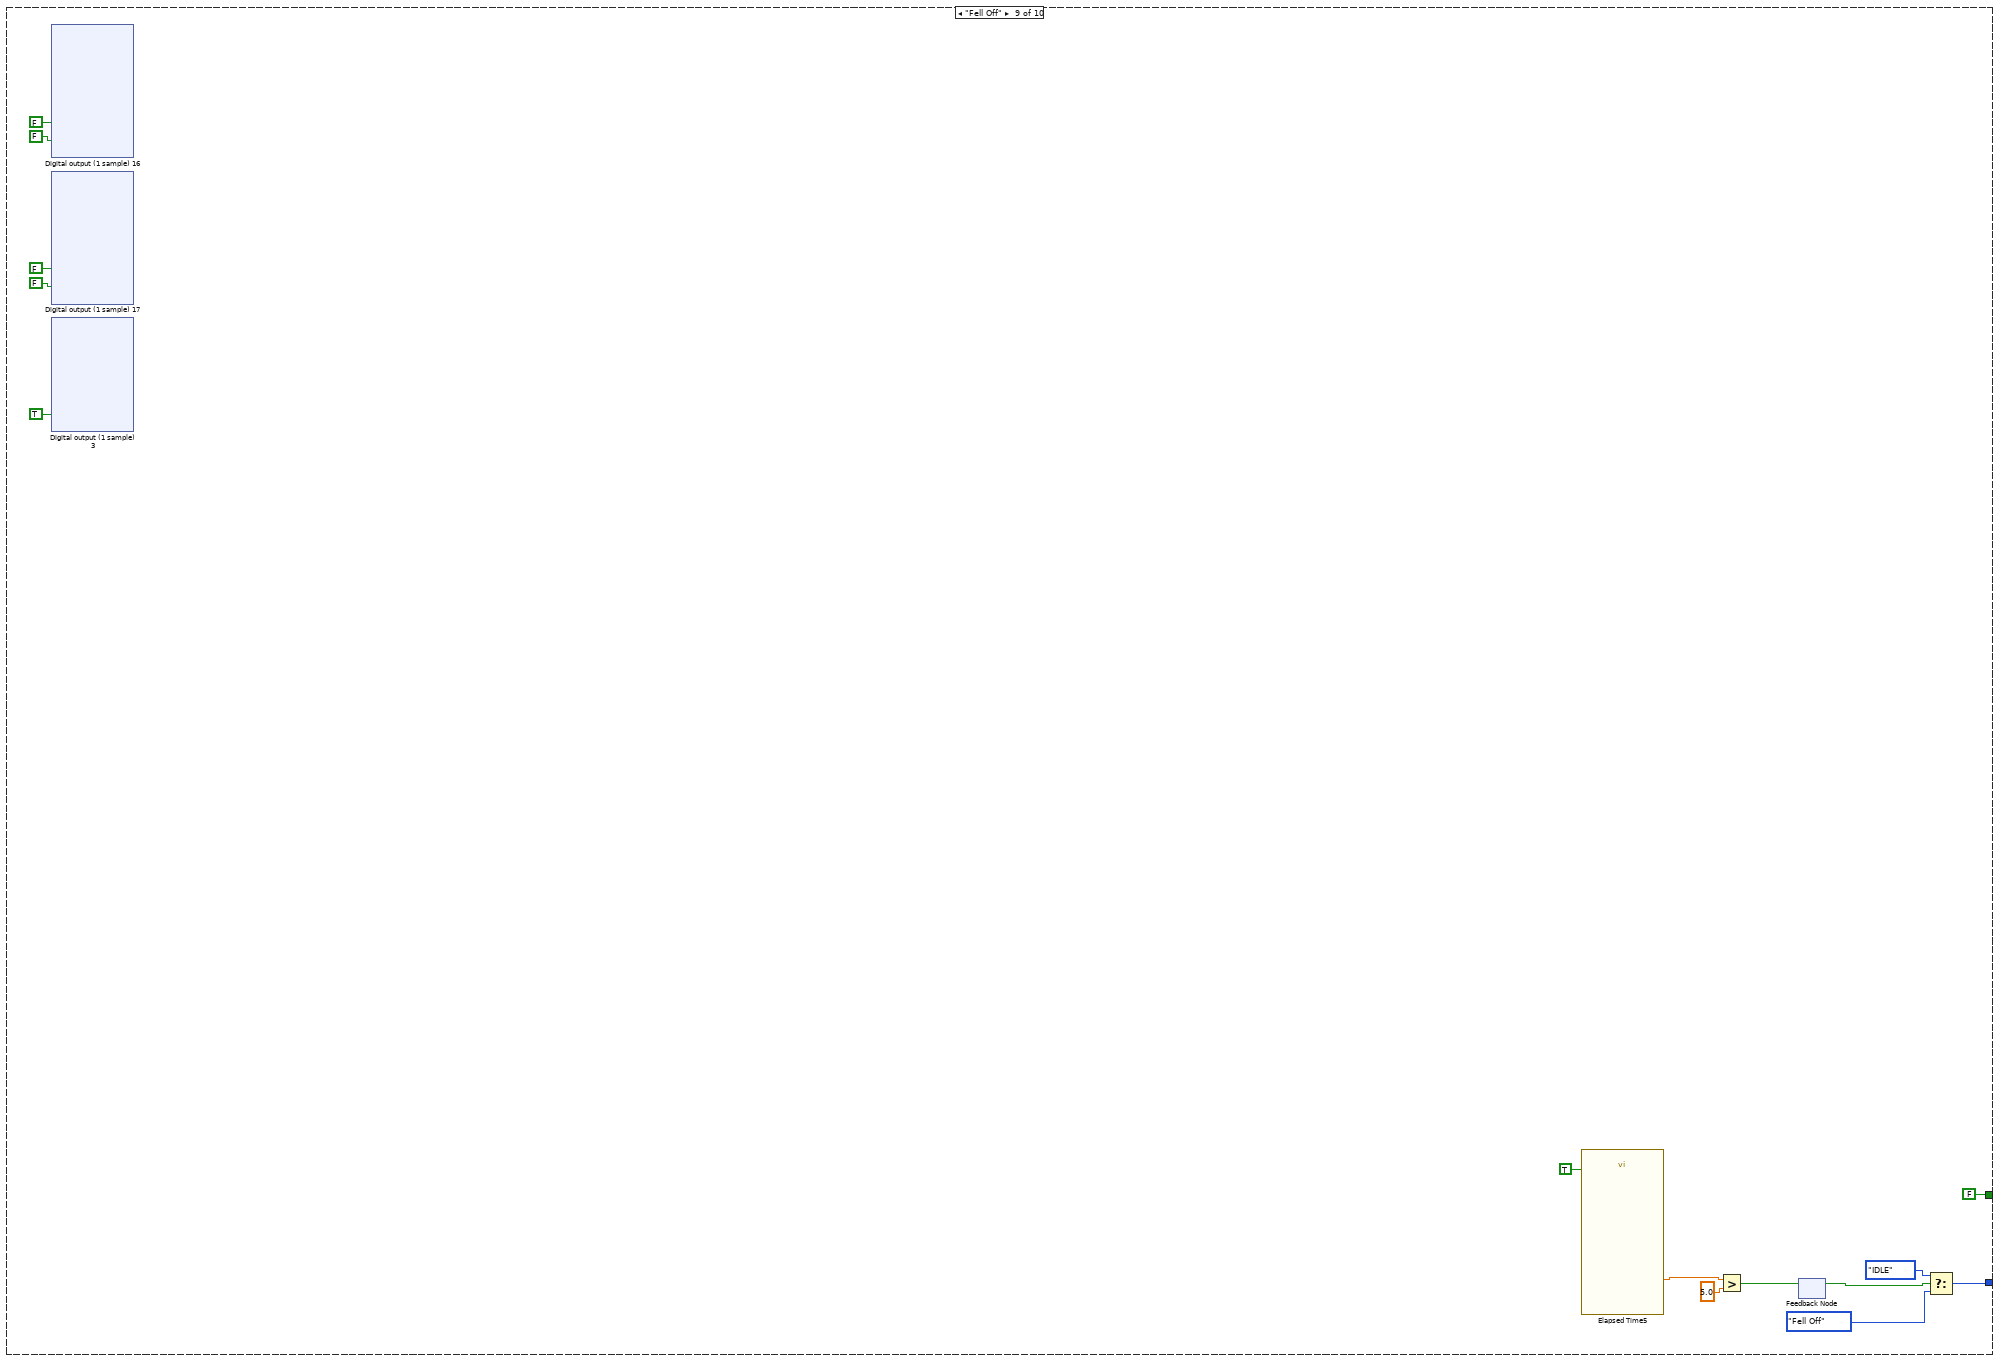
[diagram p15: hidden frame]
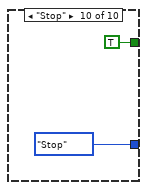
[diagram p16: hidden frame]
diagram:
  n1 = while {
    shift-right: [w26] -> _
    shift-left: T1."Turn ON" ("Enum") -> [w30]
    tunnel: [0.0 ("Duty Cycle")] -> w8
    tunnel: [0.0 ("Duty Cycle")] -> w7
    tunnel: [0.0 ("Duty Cycle")] -> w6
    tunnel: [FALSE ("A/DIO1 (Pin 13)")] -> w5
    tunnel: [FALSE ("A/DIO0 (Pin 11)")] -> w4
    tunnel: [FALSE ("A/DIO3 (Pin 17)")] -> w3
    tunnel: [FALSE ("A/DIO2 (Pin 15)")] -> w2
    tunnel: [0.0 ("Duty Cycle")] -> w1
    stop <- w19 stop-if-true
    w23 = FALSE ("Watering")
    w24 = FALSE ("Drill Down")
    n2 = invoke on="Start Farming" class="Bool" method="Reinit To Default"() -> ()  [unwired: 3 in, 3 out]
    n3 = case shown="\"Seeding\"" w30 {
      tunnel: [w36 w88 w171 w267 w470 w966 w1899 w2422 w2679 T1."Stop" ("Enum")] -> w26
      tunnel: [FALSE FALSE FALSE FALSE FALSE FALSE FALSE FALSE FALSE TRUE] -> w18
      frame "Turn ON" {
        n4 = call "Elapsed Time2"() -> ("Elapsed Time (s)"=w35:dbl)  [unwired: 12 in, 7 out]
        n5 = local write "Message"("Initializing" ("Message")) -> ()
        n6 = Less Or Equal?(x=w35, y=0.5) -> (x <= y?=w33:bool)
        n7 = local write "Intialize"(w33) -> ()
        n8 = xnode "LED"("LED0"=w33, "LED1"=w33, "LED2"=w33, "LED3"=w33) -> ()  [unwired: 1 in, 1 out]
        n9 = case shown="True" w33 {
          frame False {
          }
          frame True {
            n10 = local write "Message"("Initializing" ("Message")) -> ()
          }
        }
        n11 = feedback #1() -> (w39:bool)  [unwired: 1 in]
        n12 = call "Elapsed Time"("Reset"=w39) -> ("Elapsed Time (s)"=w42:dbl)  [unwired: 11 in, 7 out]
        n13 = Select(t=T1."IDLE" ("Enum"), s=w39, f=T1."Turn ON" ("Enum")) -> (s? t:f=w36:T1)
        n14 = Greater?(x=w42, y=3.0) -> (0:w40:bool)
        n15 = feedback-in #1(w40) -> ()
      }
      frame "IDLE", Default {
        n16 = xnode "Digital output (1 sample) 18"("A/DIO0 (Pin 11)"=FALSE, "A/DIO1 (Pin 13)"=FALSE) -> ()  [unwired: 1 in, 1 out]
        n17 = xnode "Digital output (1 sample) 19"("A/DIO2 (Pin 15)"=FALSE, "A/DIO3 (Pin 17)"=FALSE) -> ()  [unwired: 1 in, 1 out]
        n18 = local write "Message"("Waiting for Orders Sensei" ("Message")) -> ()
        n19 = local write "Switching\nMode"("Start Farming") -> ()
        n20 = case shown="True" "Start Farming" {
          tunnel: [T1."IDLE" ("Enum") T1."Start Farming" ("Enum")] -> w88
          frame False {
          }
          frame True {
          }
        }
      }
      frame "Start Farming" {
        n21 = xnode "Digital output (1 sample) 10"("A/DIO0 (Pin 11)"=FALSE, "A/DIO1 (Pin 13)"=FALSE) -> ()  [unwired: 1 in, 1 out]
        n22 = xnode "Digital output (1 sample) 11"("A/DIO2 (Pin 15)"=FALSE, "A/DIO3 (Pin 17)"=FALSE) -> ()  [unwired: 1 in, 1 out]
        n23 = local write "Message"("lets Farm" ("Message")) -> ()
        n24 = feedback #2() -> (w170:bool)  [unwired: 1 in]
        n25 = call "Elapsed Time3"("Reset"=w170) -> ("Elapsed Time (s)"=w176:dbl)  [unwired: 11 in, 7 out]
        n26 = local write "Switching\nMode"(w170) -> ()
        n27 = Select(t=T1."Drive" ("Enum"), s=w170, f=T1."Start Farming" ("Enum")) -> (s? t:f=w171:T1)
        n28 = Greater?(x=w176, y=2.0) -> (0:w174:bool)
        n29 = feedback-in #2(w174) -> ()
      }
      frame "Drive" {
        n30 = flat-sequence {
          frame #0 {
            n31 = xnode "Digital output (1 sample) 2"("A/DIO2 (Pin 15)"=TRUE, "A/DIO3 (Pin 17)"=FALSE) -> ()  [unwired: 1 in, 1 out]
            n32 = xnode "Digital output (1 sample)"("A/DIO0 (Pin 11)"=TRUE, "A/DIO1 (Pin 13)"=FALSE) -> ()  [unwired: 1 in, 1 out]
          }
        }
        n33 = xnode "PWM 11"("Duty Cycle"=0.5) -> ()  [unwired: 1 in, 1 out]
        n34 = xnode "PWM"("Duty Cycle"=0.5) -> ()  [unwired: 1 in, 1 out]
        n35 = local write "Message"("Drive forward" ("Message")) -> ()
        n36 = xnode "Accelerometer"() -> ("X-Axis"=w274:dbl, "Y-Axis"=w262:dbl)  [unwired: 1 in, 2 out]
        n37 = Greater Or Equal?(x=w274, y=0.4) -> (x >= y?=w271:bool)
        n38 = Greater Or Equal?(x=w262, y=0.4) -> (x >= y?=w264:bool)
        n39 = Less Or Equal?(x=w274, y=-0.4) -> (x <= y?=w270:bool)
        n40 = Less Or Equal?(x=w262, y=-0.4) -> (x <= y?=w263:bool)
        n41 = call "Elapsed Time4"("Reset"=TRUE) -> ("Elapsed Time (s)"=w250:dbl)  [unwired: 11 in, 7 out]
        n42 = Or(x=w271, y=w270) -> (x .or. y?=w269:bool)
        n43 = Or(x=w264, y=w263) -> (x .or. y?=w268:bool)
        n44 = Greater?(x=w250, y=2.0) -> (0:w254:bool)
        n45 = Select(t=T1."Drilling" ("Enum"), s=w254, f=T1."Drive" ("Enum")) -> (s? t:f=w249:T1)
        n46 = Or(x=w269, y=w268) -> (x .or. y?=w261:bool)
        n47 = Select(t=T1."Fell Off" ("Enum"), s=w261, f=w249) -> (s? t:f=w267:T1)
        n48 = local write "Switching\nMode"(w261) -> ()
      }
      frame "Drilling" {
        n49 = xnode "Digital output (1 sample) 8"("A/DIO0 (Pin 11)"=FALSE, "A/DIO1 (Pin 13)"=FALSE) -> ()  [unwired: 1 in, 1 out]
        n50 = xnode "Digital output (1 sample) 9"("A/DIO2 (Pin 15)"=FALSE, "A/DIO3 (Pin 17)"=FALSE) -> ()  [unwired: 1 in, 1 out]
        n51 = case shown="True" TRUE {
          frame False {
            n52 = flat-sequence {
              tunnel: u32 5 ("milliseconds to wait") -> [w497]
              tunnel: [w497] -> w492
              tunnel: [w540] -> w491
              tunnel: w492 -> [w540]
              tunnel: [w583] -> w490
              tunnel: w491 -> [w583]
              tunnel: w490 -> [w626]
              frame #0 {
                n53 = Wait (ms)(milliseconds to wait=w497) -> ()  [unwired: 1 out]
                n54 = xnode "Digital output (1 sample) 24"("B/DIO0 (Pin 11)"=TRUE, "B/DIO1 (Pin 13)"=FALSE, "B/DIO2 (Pin 15)"=FALSE, "B/DIO3 (Pin 17)"=FALSE) -> ()  [unwired: 1 in, 1 out]
              }
              frame #1 {
                n55 = Wait (ms)(milliseconds to wait=w540) -> ()  [unwired: 1 out]
                n56 = xnode "Digital output (1 sample) 25"("B/DIO0 (Pin 11)"=FALSE, "B/DIO1 (Pin 13)"=TRUE, "B/DIO2 (Pin 15)"=FALSE, "B/DIO3 (Pin 17)"=FALSE) -> ()  [unwired: 1 in, 1 out]
              }
              frame #2 {
                n57 = Wait (ms)(milliseconds to wait=w583) -> ()  [unwired: 1 out]
                n58 = xnode "Digital output (1 sample) 26"("B/DIO0 (Pin 11)"=FALSE, "B/DIO1 (Pin 13)"=FALSE, "B/DIO2 (Pin 15)"=TRUE, "B/DIO3 (Pin 17)"=FALSE) -> ()  [unwired: 1 in, 1 out]
              }
              frame #3 {
                n59 = Wait (ms)(milliseconds to wait=w626) -> ()  [unwired: 1 out]
                n60 = xnode "Digital output (1 sample) 27"("B/DIO0 (Pin 11)"=FALSE, "B/DIO1 (Pin 13)"=FALSE, "B/DIO2 (Pin 15)"=FALSE, "B/DIO3 (Pin 17)"=TRUE) -> ()  [unwired: 1 in, 1 out]
              }
            }
          }
          frame True {
            n61 = flat-sequence {
              tunnel: u32 5 ("milliseconds to wait") -> [w673]
              tunnel: [w673] -> w665
              tunnel: [w716] -> w666
              tunnel: w665 -> [w716]
              tunnel: [w759] -> w667
              tunnel: w666 -> [w759]
              tunnel: w667 -> [w802]
              frame #0 {
                n62 = Wait (ms)(milliseconds to wait=w673) -> ()  [unwired: 1 out]
                n63 = xnode "Digital output (1 sample) 20"("B/DIO0 (Pin 11)"=FALSE, "B/DIO1 (Pin 13)"=FALSE, "B/DIO2 (Pin 15)"=FALSE, "B/DIO3 (Pin 17)"=TRUE) -> ()  [unwired: 1 in, 1 out]
              }
              frame #1 {
                n64 = Wait (ms)(milliseconds to wait=w716) -> ()  [unwired: 1 out]
                n65 = xnode "Digital output (1 sample) 21"("B/DIO0 (Pin 11)"=FALSE, "B/DIO1 (Pin 13)"=FALSE, "B/DIO2 (Pin 15)"=TRUE, "B/DIO3 (Pin 17)"=FALSE) -> ()  [unwired: 1 in, 1 out]
              }
              frame #2 {
                n66 = Wait (ms)(milliseconds to wait=w759) -> ()  [unwired: 1 out]
                n67 = xnode "Digital output (1 sample) 22"("B/DIO0 (Pin 11)"=FALSE, "B/DIO1 (Pin 13)"=TRUE, "B/DIO2 (Pin 15)"=FALSE, "B/DIO3 (Pin 17)"=FALSE) -> ()  [unwired: 1 in, 1 out]
              }
              frame #3 {
                n68 = Wait (ms)(milliseconds to wait=w802) -> ()  [unwired: 1 out]
                n69 = xnode "Digital output (1 sample) 23"("B/DIO0 (Pin 11)"=TRUE, "B/DIO1 (Pin 13)"=FALSE, "B/DIO2 (Pin 15)"=FALSE, "B/DIO3 (Pin 17)"=FALSE) -> ()  [unwired: 1 in, 1 out]
              }
            }
          }
        }
        n70 = local write "Message"("Drilling the hole" ("Message")) -> ()
        n71 = xnode "Accelerometer 2"() -> ("X-Axis"=w484:dbl, "Y-Axis"=w471:dbl)  [unwired: 1 in, 2 out]
        n72 = call "Elapsed Time6"("Reset"=TRUE) -> ("Elapsed Time (s)"=w488:dbl)  [unwired: 11 in, 7 out]
        n73 = Greater Or Equal?(x=w484, y=0.4) -> (x >= y?=w481:bool)
        n74 = Greater Or Equal?(x=w471, y=0.4) -> (x >= y?=w473:bool)
        n75 = Less Or Equal?(x=w484, y=-0.4) -> (x <= y?=w480:bool)
        n76 = Less Or Equal?(x=w471, y=-0.4) -> (x <= y?=w472:bool)
        n77 = Or(x=w481, y=w480) -> (x .or. y?=w479:bool)
        n78 = Or(x=w473, y=w472) -> (x .or. y?=w478:bool)
        n79 = Greater?(x=w488, y=4.0) -> (0:w460:bool)
        n80 = Select(t=T1."Seeding" ("Enum"), s=w460, f=T1."Drilling" ("Enum")) -> (s? t:f=w476:T1)
        n81 = Or(x=w479, y=w478) -> (x .or. y?=w469:bool)
        n82 = local write "Switching\nMode"(w469) -> ()
        n83 = Select(t=T1."Fell Off" ("Enum"), s=w469, f=w476) -> (s? t:f=w470:T1)
      }
      frame "Seeding" {
        n84 = flat-sequence {
          frame #0 {
            w1410 = 60.0 ("servo 1")
            n85 = Wait (ms)(milliseconds to wait=u32 3000) -> ()  [unwired: 1 out]
            n86 = local write "Angle 1"(w1410) -> ()
            n87 = call <vilib>:"Polynomial Interpolation.vi"("x value"=w1410, "X"=dbl[] [0.0, 180.0], "Y"=dbl[] [0.15, 0.03]) -> ("interpolation value"=w1412:dbl)  [unwired: 2 out]
            n88 = xnode "PWM 4"("Duty Cycle"=w1412) -> ()  [unwired: 1 in, 1 out]
            n89 = Divide(x=1.0, y=50.0) -> (x/y=w1411:dbl)
            n90 = Multiply(x=w1412, y=w1411) -> (x*y=w1413:dbl)
            n91 = local write "pulse width 1"(w1413) -> ()
          }
          frame #1 {
            w1453 = 60.0 ("servo 1")
            n92 = local write "Angle 2"(w1453) -> ()
            n93 = call <vilib>:"Polynomial Interpolation.vi"("x value"=w1453, "X"=dbl[] [0.0, 180.0], "Y"=dbl[] [0.15, 0.03]) -> ("interpolation value"=w1455:dbl)  [unwired: 2 out]
            n94 = xnode "PWM 5"("Duty Cycle"=w1455) -> ()  [unwired: 1 in, 1 out]
            n95 = Divide(x=1.0, y=50.0) -> (x/y=w1454:dbl)
            n96 = Multiply(x=w1455, y=w1454) -> (x*y=w1456:dbl)
            n97 = local write "pulse width 2"(w1456) -> ()
          }
          frame #2 {
            n98 = case shown="True" TRUE {
              frame False {
                n99 = flat-sequence {
                  tunnel: u32 5 ("milliseconds to wait") -> [w1501]
                  tunnel: [w1501] -> w1496
                  tunnel: [w1544] -> w1495
                  tunnel: w1496 -> [w1544]
                  tunnel: [w1587] -> w1494
                  tunnel: w1495 -> [w1587]
                  tunnel: w1494 -> [w1630]
                  frame #0 {
                    n100 = Wait (ms)(milliseconds to wait=w1501) -> ()  [unwired: 1 out]
                    n101 = xnode "Digital output (1 sample) 28"("B/DIO4 (Pin 19)"=FALSE ("B/DIO0 (Pin 11)"), "B/DIO5 (Pin 21)"=FALSE ("B/DIO1 (Pin 13)"), "B/DIO6 (Pin 23)"=FALSE ("B/DIO2 (Pin 15)"), "B/DIO7 (Pin 25)"=TRUE ("B/DIO3 (Pin 17)")) -> ()  [unwired: 1 in, 1 out]
                  }
                  frame #1 {
                    n102 = Wait (ms)(milliseconds to wait=w1544) -> ()  [unwired: 1 out]
                    n103 = xnode "Digital output (1 sample) 29"("B/DIO4 (Pin 19)"=FALSE ("B/DIO0 (Pin 11)"), "B/DIO5 (Pin 21)"=FALSE ("B/DIO1 (Pin 13)"), "B/DIO6 (Pin 23)"=TRUE ("B/DIO2 (Pin 15)"), "B/DIO7 (Pin 25)"=FALSE ("B/DIO3 (Pin 17)")) -> ()  [unwired: 1 in, 1 out]
                  }
                  frame #2 {
                    n104 = Wait (ms)(milliseconds to wait=w1587) -> ()  [unwired: 1 out]
                    n105 = xnode "Digital output (1 sample) 30"("B/DIO4 (Pin 19)"=FALSE ("B/DIO0 (Pin 11)"), "B/DIO5 (Pin 21)"=TRUE ("B/DIO1 (Pin 13)"), "B/DIO6 (Pin 23)"=FALSE ("B/DIO2 (Pin 15)"), "B/DIO7 (Pin 25)"=FALSE ("B/DIO3 (Pin 17)")) -> ()  [unwired: 1 in, 1 out]
                  }
                  frame #3 {
                    n106 = Wait (ms)(milliseconds to wait=w1630) -> ()  [unwired: 1 out]
                    n107 = xnode "Digital output (1 sample) 31"("B/DIO4 (Pin 19)"=TRUE ("B/DIO0 (Pin 11)"), "B/DIO5 (Pin 21)"=FALSE ("B/DIO1 (Pin 13)"), "B/DIO6 (Pin 23)"=FALSE ("B/DIO2 (Pin 15)"), "B/DIO7 (Pin 25)"=FALSE ("B/DIO3 (Pin 17)")) -> ()  [unwired: 1 in, 1 out]
                  }
                }
              }
              frame True {
                n108 = flat-sequence {
                  tunnel: u32 5 ("milliseconds to wait") -> [w1677]
                  tunnel: [w1677] -> w1669
                  tunnel: [w1720] -> w1670
                  tunnel: w1669 -> [w1720]
                  tunnel: [w1763] -> w1671
                  tunnel: w1670 -> [w1763]
                  tunnel: w1671 -> [w1806]
                  frame #0 {
                    n109 = Wait (ms)(milliseconds to wait=w1677) -> ()  [unwired: 1 out]
                    n110 = xnode "Digital output (1 sample) 32"("B/DIO4 (Pin 19)"=TRUE ("B/DIO0 (Pin 11)"), "B/DIO5 (Pin 21)"=FALSE ("B/DIO1 (Pin 13)"), "B/DIO6 (Pin 23)"=FALSE ("B/DIO2 (Pin 15)"), "B/DIO7 (Pin 25)"=FALSE ("B/DIO3 (Pin 17)")) -> ()  [unwired: 1 in, 1 out]
                  }
                  frame #1 {
                    n111 = Wait (ms)(milliseconds to wait=w1720) -> ()  [unwired: 1 out]
                    n112 = xnode "Digital output (1 sample) 33"("B/DIO4 (Pin 19)"=FALSE ("B/DIO0 (Pin 11)"), "B/DIO5 (Pin 21)"=TRUE ("B/DIO1 (Pin 13)"), "B/DIO6 (Pin 23)"=FALSE ("B/DIO2 (Pin 15)"), "B/DIO7 (Pin 25)"=FALSE ("B/DIO3 (Pin 17)")) -> ()  [unwired: 1 in, 1 out]
                  }
                  frame #2 {
                    n113 = Wait (ms)(milliseconds to wait=w1763) -> ()  [unwired: 1 out]
                    n114 = xnode "Digital output (1 sample) 34"("B/DIO4 (Pin 19)"=FALSE ("B/DIO0 (Pin 11)"), "B/DIO5 (Pin 21)"=FALSE ("B/DIO1 (Pin 13)"), "B/DIO6 (Pin 23)"=TRUE ("B/DIO2 (Pin 15)"), "B/DIO7 (Pin 25)"=FALSE ("B/DIO3 (Pin 17)")) -> ()  [unwired: 1 in, 1 out]
                  }
                  frame #3 {
                    n115 = Wait (ms)(milliseconds to wait=w1806) -> ()  [unwired: 1 out]
                    n116 = xnode "Digital output (1 sample) 35"("B/DIO4 (Pin 19)"=FALSE ("B/DIO0 (Pin 11)"), "B/DIO5 (Pin 21)"=FALSE ("B/DIO1 (Pin 13)"), "B/DIO6 (Pin 23)"=FALSE ("B/DIO2 (Pin 15)"), "B/DIO7 (Pin 25)"=TRUE ("B/DIO3 (Pin 17)")) -> ()  [unwired: 1 in, 1 out]
                  }
                }
              }
            }
          }
        }
        n117 = xnode "Digital output (1 sample) 12"("A/DIO0 (Pin 11)"=FALSE, "A/DIO1 (Pin 13)"=FALSE) -> ()  [unwired: 1 in, 1 out]
        n118 = xnode "Digital output (1 sample) 13"("A/DIO2 (Pin 15)"=FALSE, "A/DIO3 (Pin 17)"=FALSE) -> ()  [unwired: 1 in, 1 out]
        n119 = case shown="False" FALSE {
          frame False {
            n120 = flat-sequence {
              tunnel: u32 5 ("milliseconds to wait") -> [w1061]
              tunnel: [w1061] -> w1056
              tunnel: [w1104] -> w1055
              tunnel: w1056 -> [w1104]
              tunnel: [w1147] -> w1054
              tunnel: w1055 -> [w1147]
              tunnel: w1054 -> [w1190]
              frame #0 {
                n121 = Wait (ms)(milliseconds to wait=w1061) -> ()  [unwired: 1 out]
                n122 = xnode "Digital output (1 sample) 36"("B/DIO0 (Pin 11)"=TRUE, "B/DIO1 (Pin 13)"=FALSE, "B/DIO2 (Pin 15)"=FALSE, "B/DIO3 (Pin 17)"=FALSE) -> ()  [unwired: 1 in, 1 out]
              }
              frame #1 {
                n123 = Wait (ms)(milliseconds to wait=w1104) -> ()  [unwired: 1 out]
                n124 = xnode "Digital output (1 sample) 37"("B/DIO0 (Pin 11)"=FALSE, "B/DIO1 (Pin 13)"=TRUE, "B/DIO2 (Pin 15)"=FALSE, "B/DIO3 (Pin 17)"=FALSE) -> ()  [unwired: 1 in, 1 out]
              }
              frame #2 {
                n125 = Wait (ms)(milliseconds to wait=w1147) -> ()  [unwired: 1 out]
                n126 = xnode "Digital output (1 sample) 38"("B/DIO0 (Pin 11)"=FALSE, "B/DIO1 (Pin 13)"=FALSE, "B/DIO2 (Pin 15)"=TRUE, "B/DIO3 (Pin 17)"=FALSE) -> ()  [unwired: 1 in, 1 out]
              }
              frame #3 {
                n127 = Wait (ms)(milliseconds to wait=w1190) -> ()  [unwired: 1 out]
                n128 = xnode "Digital output (1 sample) 39"("B/DIO0 (Pin 11)"=FALSE, "B/DIO1 (Pin 13)"=FALSE, "B/DIO2 (Pin 15)"=FALSE, "B/DIO3 (Pin 17)"=TRUE) -> ()  [unwired: 1 in, 1 out]
              }
            }
          }
          frame True {
            n129 = flat-sequence {
              tunnel: u32 5 ("milliseconds to wait") -> [w1237]
              tunnel: [w1237] -> w1229
              tunnel: [w1280] -> w1230
              tunnel: w1229 -> [w1280]
              tunnel: [w1323] -> w1231
              tunnel: w1230 -> [w1323]
              tunnel: w1231 -> [w1366]
              frame #0 {
                n130 = Wait (ms)(milliseconds to wait=w1237) -> ()  [unwired: 1 out]
                n131 = xnode "Digital output (1 sample) 40"("B/DIO0 (Pin 11)"=FALSE, "B/DIO1 (Pin 13)"=FALSE, "B/DIO2 (Pin 15)"=FALSE, "B/DIO3 (Pin 17)"=TRUE) -> ()  [unwired: 1 in, 1 out]
              }
              frame #1 {
                n132 = Wait (ms)(milliseconds to wait=w1280) -> ()  [unwired: 1 out]
                n133 = xnode "Digital output (1 sample) 41"("B/DIO0 (Pin 11)"=FALSE, "B/DIO1 (Pin 13)"=FALSE, "B/DIO2 (Pin 15)"=TRUE, "B/DIO3 (Pin 17)"=FALSE) -> ()  [unwired: 1 in, 1 out]
              }
              frame #2 {
                n134 = Wait (ms)(milliseconds to wait=w1323) -> ()  [unwired: 1 out]
                n135 = xnode "Digital output (1 sample) 42"("B/DIO0 (Pin 11)"=FALSE, "B/DIO1 (Pin 13)"=TRUE, "B/DIO2 (Pin 15)"=FALSE, "B/DIO3 (Pin 17)"=FALSE) -> ()  [unwired: 1 in, 1 out]
              }
              frame #3 {
                n136 = Wait (ms)(milliseconds to wait=w1366) -> ()  [unwired: 1 out]
                n137 = xnode "Digital output (1 sample) 43"("B/DIO0 (Pin 11)"=TRUE, "B/DIO1 (Pin 13)"=FALSE, "B/DIO2 (Pin 15)"=FALSE, "B/DIO3 (Pin 17)"=FALSE) -> ()  [unwired: 1 in, 1 out]
              }
            }
          }
        }
        n138 = local write "Message"("Seeding" ("Message")) -> ()
        n139 = xnode "Accelerometer 3"() -> ("X-Axis"=w980:dbl, "Y-Axis"=w968:dbl)  [unwired: 1 in, 2 out]
        n140 = call "Elapsed Time7"("Reset"=TRUE) -> ("Elapsed Time (s)"=w961:dbl)  [unwired: 11 in, 7 out]
        n141 = Greater Or Equal?(x=w980, y=0.4) -> (x >= y?=w977:bool)
        n142 = Greater Or Equal?(x=w968, y=0.4) -> (x >= y?=w970:bool)
        n143 = Less Or Equal?(x=w980, y=-0.4) -> (x <= y?=w976:bool)
        n144 = Less Or Equal?(x=w968, y=-0.4) -> (x <= y?=w969:bool)
        n145 = Or(x=w977, y=w976) -> (x .or. y?=w975:bool)
        n146 = Or(x=w970, y=w969) -> (x .or. y?=w974:bool)
        n147 = Greater?(x=w961, y=4.0) -> (0:w962:bool)
        n148 = Select(t=T1."Watering" ("Enum"), s=w962, f=T1."Seeding" ("Enum")) -> (s? t:f=w956:T1)
        n149 = Or(x=w975, y=w974) -> (x .or. y?=w967:bool)
        n150 = local write "Switching\nMode"(w967) -> ()
        n151 = Select(t=T1."Fell Off" ("Enum"), s=w967, f=w956) -> (s? t:f=w966:T1)
      }
      frame "Watering" {
        w1890 = 60.0 ("servo 1")
        n152 = flat-sequence {
          frame #0 {
            n153 = case shown="False" FALSE {
              frame False {
                n154 = flat-sequence {
                  tunnel: u32 5 ("milliseconds to wait") -> [w1928]
                  tunnel: [w1928] -> w1923
                  tunnel: [w1971] -> w1922
                  tunnel: w1923 -> [w1971]
                  tunnel: [w2014] -> w1921
                  tunnel: w1922 -> [w2014]
                  tunnel: w1921 -> [w2057]
                  frame #0 {
                    n155 = Wait (ms)(milliseconds to wait=w1928) -> ()  [unwired: 1 out]
                    n156 = xnode "Digital output (1 sample) 44"("B/DIO4 (Pin 19)"=FALSE ("B/DIO0 (Pin 11)"), "B/DIO5 (Pin 21)"=FALSE ("B/DIO1 (Pin 13)"), "B/DIO6 (Pin 23)"=FALSE ("B/DIO2 (Pin 15)"), "B/DIO7 (Pin 25)"=TRUE ("B/DIO3 (Pin 17)")) -> ()  [unwired: 1 in, 1 out]
                  }
                  frame #1 {
                    n157 = Wait (ms)(milliseconds to wait=w1971) -> ()  [unwired: 1 out]
                    n158 = xnode "Digital output (1 sample) 45"("B/DIO4 (Pin 19)"=FALSE ("B/DIO0 (Pin 11)"), "B/DIO5 (Pin 21)"=FALSE ("B/DIO1 (Pin 13)"), "B/DIO6 (Pin 23)"=TRUE ("B/DIO2 (Pin 15)"), "B/DIO7 (Pin 25)"=FALSE ("B/DIO3 (Pin 17)")) -> ()  [unwired: 1 in, 1 out]
                  }
                  frame #2 {
                    n159 = Wait (ms)(milliseconds to wait=w2014) -> ()  [unwired: 1 out]
                    n160 = xnode "Digital output (1 sample) 46"("B/DIO4 (Pin 19)"=FALSE ("B/DIO0 (Pin 11)"), "B/DIO5 (Pin 21)"=TRUE ("B/DIO1 (Pin 13)"), "B/DIO6 (Pin 23)"=FALSE ("B/DIO2 (Pin 15)"), "B/DIO7 (Pin 25)"=FALSE ("B/DIO3 (Pin 17)")) -> ()  [unwired: 1 in, 1 out]
                  }
                  frame #3 {
                    n161 = Wait (ms)(milliseconds to wait=w2057) -> ()  [unwired: 1 out]
                    n162 = xnode "Digital output (1 sample) 47"("B/DIO4 (Pin 19)"=TRUE ("B/DIO0 (Pin 11)"), "B/DIO5 (Pin 21)"=FALSE ("B/DIO1 (Pin 13)"), "B/DIO6 (Pin 23)"=FALSE ("B/DIO2 (Pin 15)"), "B/DIO7 (Pin 25)"=FALSE ("B/DIO3 (Pin 17)")) -> ()  [unwired: 1 in, 1 out]
                  }
                }
              }
              frame True {
                n163 = flat-sequence {
                  tunnel: u32 5 ("milliseconds to wait") -> [w2104]
                  tunnel: [w2104] -> w2096
                  tunnel: [w2147] -> w2097
                  tunnel: w2096 -> [w2147]
                  tunnel: [w2190] -> w2098
                  tunnel: w2097 -> [w2190]
                  tunnel: w2098 -> [w2233]
                  frame #0 {
                    n164 = Wait (ms)(milliseconds to wait=w2104) -> ()  [unwired: 1 out]
                    n165 = xnode "Digital output (1 sample) 48"("B/DIO4 (Pin 19)"=TRUE ("B/DIO0 (Pin 11)"), "B/DIO5 (Pin 21)"=FALSE ("B/DIO1 (Pin 13)"), "B/DIO6 (Pin 23)"=FALSE ("B/DIO2 (Pin 15)"), "B/DIO7 (Pin 25)"=FALSE ("B/DIO3 (Pin 17)")) -> ()  [unwired: 1 in, 1 out]
                  }
                  frame #1 {
                    n166 = Wait (ms)(milliseconds to wait=w2147) -> ()  [unwired: 1 out]
                    n167 = xnode "Digital output (1 sample) 49"("B/DIO4 (Pin 19)"=FALSE ("B/DIO0 (Pin 11)"), "B/DIO5 (Pin 21)"=TRUE ("B/DIO1 (Pin 13)"), "B/DIO6 (Pin 23)"=FALSE ("B/DIO2 (Pin 15)"), "B/DIO7 (Pin 25)"=FALSE ("B/DIO3 (Pin 17)")) -> ()  [unwired: 1 in, 1 out]
                  }
                  frame #2 {
                    n168 = Wait (ms)(milliseconds to wait=w2190) -> ()  [unwired: 1 out]
                    n169 = xnode "Digital output (1 sample) 50"("B/DIO4 (Pin 19)"=FALSE ("B/DIO0 (Pin 11)"), "B/DIO5 (Pin 21)"=FALSE ("B/DIO1 (Pin 13)"), "B/DIO6 (Pin 23)"=TRUE ("B/DIO2 (Pin 15)"), "B/DIO7 (Pin 25)"=FALSE ("B/DIO3 (Pin 17)")) -> ()  [unwired: 1 in, 1 out]
                  }
                  frame #3 {
                    n170 = Wait (ms)(milliseconds to wait=w2233) -> ()  [unwired: 1 out]
                    n171 = xnode "Digital output (1 sample) 51"("B/DIO4 (Pin 19)"=FALSE ("B/DIO0 (Pin 11)"), "B/DIO5 (Pin 21)"=FALSE ("B/DIO1 (Pin 13)"), "B/DIO6 (Pin 23)"=FALSE ("B/DIO2 (Pin 15)"), "B/DIO7 (Pin 25)"=TRUE ("B/DIO3 (Pin 17)")) -> ()  [unwired: 1 in, 1 out]
                  }
                }
              }
            }
          }
        }
        n172 = xnode "Digital output (1 sample) 14"("A/DIO0 (Pin 11)"=FALSE, "A/DIO1 (Pin 13)"=FALSE) -> ()  [unwired: 1 in, 1 out]
        n173 = xnode "Digital output (1 sample) 15"("A/DIO2 (Pin 15)"=FALSE, "A/DIO3 (Pin 17)"=FALSE) -> ()  [unwired: 1 in, 1 out]
        n174 = local write "Angle 1"(w1890) -> ()
        n175 = call <vilib>:"Polynomial Interpolation.vi"("x value"=w1890, "X"=dbl[] [0.0, 180.0], "Y"=dbl[] [0.15, 0.03]) -> ("interpolation value"=w1893:dbl)  [unwired: 2 out]
        n176 = xnode "PWM 6"("Duty Cycle"=w1893) -> ()  [unwired: 1 in, 1 out]
        n177 = Divide(x=1.0, y=50.0) -> (x/y=w1894:dbl)
        n178 = Multiply(x=w1893, y=w1894) -> (x*y=w1892:dbl)
        n179 = local write "pulse width 1"(w1892) -> ()
        n180 = xnode "Accelerometer 4"() -> ("X-Axis"=w1914:dbl, "Y-Axis"=w1901:dbl)  [unwired: 1 in, 2 out]
        n181 = call "Elapsed Time8"("Reset"=TRUE) -> ("Elapsed Time (s)"=w1918:dbl)  [unwired: 11 in, 7 out]
        n182 = Greater Or Equal?(x=w1914, y=0.4) -> (x >= y?=w1911:bool)
        n183 = Greater Or Equal?(x=w1901, y=0.4) -> (x >= y?=w1903:bool)
        n184 = Less Or Equal?(x=w1914, y=-0.4) -> (x <= y?=w1910:bool)
        n185 = Less Or Equal?(x=w1901, y=-0.4) -> (x <= y?=w1902:bool)
        n186 = Or(x=w1911, y=w1910) -> (x .or. y?=w1909:bool)
        n187 = Or(x=w1903, y=w1902) -> (x .or. y?=w1908:bool)
        n188 = Greater?(x=w1918, y=10.0) -> (0:w1885:bool)
        n189 = Select(t=T1."Filling" ("Enum"), s=w1885, f=T1."Watering" ("Enum")) -> (s? t:f=w1906:T1)
        n190 = Or(x=w1909, y=w1908) -> (x .or. y?=w1900:bool)
        n191 = local write "Switching\nMode"(w1900) -> ()
        n192 = Select(t=T1."Fell Off" ("Enum"), s=w1900, f=w1906) -> (s? t:f=w1899:T1)
      }
      frame "Filling" {
        n193 = flat-sequence {
          frame #0 {
            n194 = xnode "Digital output (1 sample) 4"("A/DIO0 (Pin 11)"=TRUE, "A/DIO1 (Pin 13)"=FALSE) -> ()  [unwired: 1 in, 1 out]
            n195 = xnode "Digital output (1 sample) 5"("A/DIO2 (Pin 15)"=TRUE, "A/DIO3 (Pin 17)"=FALSE) -> ()  [unwired: 1 in, 1 out]
          }
          frame #1 {
            w2524 = 60.0 ("servo 1")
            n196 = xnode "PWM 12"("Duty Cycle"=0.5) -> ()  [unwired: 1 in, 1 out]
            n197 = call <vilib>:"Polynomial Interpolation.vi"("x value"=w2524, "X"=dbl[] [0.0, 180.0], "Y"=dbl[] [0.15, 0.03]) -> ("interpolation value"=w2527:dbl)  [unwired: 2 out]
            n198 = local write "Angle 1"(w2524) -> ()
            n199 = xnode "PWM 7"("Duty Cycle"=w2527) -> ()  [unwired: 1 in, 1 out]
            n200 = Divide(x=1.0, y=50.0) -> (x/y=w2526:dbl)
            n201 = Multiply(x=w2527, y=w2526) -> (x*y=w2528:dbl)
            n202 = local write "pulse width 1"(w2528) -> ()
          }
        }
        n203 = xnode "PWM 3"("Duty Cycle"=0.5) -> ()  [unwired: 1 in, 1 out]
        n204 = local write "Message"("Filling the hole" ("Message")) -> ()
        n205 = xnode "Accelerometer 5"() -> ("X-Axis"=w2437:dbl, "Y-Axis"=w2424:dbl)  [unwired: 1 in, 2 out]
        n206 = call "Elapsed Time9"("Reset"=TRUE) -> ("Elapsed Time (s)"=w2443:dbl)  [unwired: 11 in, 7 out]
        n207 = Less Or Equal?(x=w2437, y=-0.4) -> (x <= y?=w2433:bool)
        n208 = Less Or Equal?(x=w2424, y=-0.4) -> (x <= y?=w2425:bool)
        n209 = Greater?(x=w2443, y=2.0) -> (0:w2441:bool)
        n210 = Greater Or Equal?(x=w2437, y=0.4) -> (x >= y?=w2434:bool)
        n211 = Greater Or Equal?(x=w2424, y=0.4) -> (x >= y?=w2426:bool)
        n212 = Or(x=w2434, y=w2433) -> (x .or. y?=w2432:bool)
        n213 = Or(x=w2426, y=w2425) -> (x .or. y?=w2431:bool)
        n214 = feedback #3() -> (w2440:bool)  [unwired: 1 in]
        n215 = feedback-in #3(w2441) -> ()
        n216 = Select(t=T1."Start Farming" ("Enum"), s=w2440, f=T1."Filling" ("Enum")) -> (s? t:f=w2429:T1)
        n217 = Or(x=w2432, y=w2431) -> (x .or. y?=w2423:bool)
        n218 = local write "Switching\nMode"(w2423) -> ()
        n219 = Select(t=T1."Fell Off" ("Enum"), s=w2423, f=w2429) -> (s? t:f=w2422:T1)
      }
      frame "Fell Off" {
        n220 = xnode "Digital output (1 sample) 16"("A/DIO0 (Pin 11)"=FALSE, "A/DIO1 (Pin 13)"=FALSE) -> ()  [unwired: 1 in, 1 out]
        n221 = xnode "Digital output (1 sample) 17"("A/DIO2 (Pin 15)"=FALSE, "A/DIO3 (Pin 17)"=FALSE) -> ()  [unwired: 1 in, 1 out]
        n222 = xnode "Digital output (1 sample) 3"("A/DIO4 (Pin 19)"=TRUE) -> ()  [unwired: 1 in, 1 out]
        n223 = call "Elapsed Time5"("Reset"=TRUE) -> ("Elapsed Time (s)"=w2686:dbl)  [unwired: 11 in, 7 out]
        n224 = Greater?(x=w2686, y=5.0) -> (0:w2684:bool)
        n225 = feedback #4() -> (w2683:bool)  [unwired: 1 in]
        n226 = feedback-in #4(w2684) -> ()
        n227 = Select(t=T1."IDLE" ("Enum"), s=w2683, f=T1."Fell Off" ("Enum")) -> (s? t:f=w2679:T1)
      }
      frame "Stop" {
      }
    }
    "State" <- w26
    n228 = local write "Intialize"(FALSE ("Intialize")) -> ()
    n229 = local write "Seeding\nUp"(FALSE ("Seeding\nUp")) -> ()
    n230 = local write "Switching\nMode"(FALSE ("Switching\nMode")) -> ()
    n231 = local write "Message"("" ("Message")) -> ()
    n232 = local write "Watering"(w23) -> ()
    n233 = local write "Drill Up"(w23) -> ()
    n234 = local write "Drill Down"(w24) -> ()
    n235 = local write "Seeding\nDown"(w24) -> ()
    n236 = Wait Until Next ms Multiple(millisecond multiple=u32 100) -> ()  [unwired: 1 out]
    n237 = Wait Until Next ms Multiple(millisecond multiple=u32 100) -> ()  [unwired: 1 out]
    n238 = Or(x=w18, y="stop") -> (x .or. y?=w19:bool)
  }
  n239 = xnode "PWM 10"("Duty Cycle"=w1) -> ()  [unwired: 1 in, 1 out]
  n240 = xnode "Digital output (1 sample) 6"("A/DIO0 (Pin 11)"=w4, "A/DIO1 (Pin 13)"=w5) -> ()  [unwired: 1 in, 1 out]
  n241 = xnode "PWM 2"("Duty Cycle"=w8) -> ()  [unwired: 1 in, 1 out]
  n242 = xnode "PWM 8"("Duty Cycle"=w7) -> ()  [unwired: 1 in, 1 out]
  n243 = xnode "Digital output (1 sample) 7"("A/DIO2 (Pin 15)"=w2, "A/DIO3 (Pin 17)"=w3) -> ()  [unwired: 1 in, 1 out]
  n244 = xnode "PWM 9"("Duty Cycle"=w6) -> ()  [unwired: 1 in, 1 out]
